vi "ME_acquire_11_DeltaForce.vi"() -> ()   [LabVIEW 2015]
doc: "Use this template to build a producer/consumer design pattern. Use this template when you need to execute a process, such as data analysis, when a data source, such as a triggered acquisition, produces data at an uneven rate and you need to execute the process when the data becomes available."
uses:
  Mode.ctl
  oxford_driver/Oxford Drivers/BUSGEN.LLB/OxfordAddress.ctl
  <vilib>/Analysis/baseanly.llb/Mean (DBL).vi
  <vilib>/Utility/file.llb/Write Delimited Spreadsheet (DBL).vi
  <vilib>/express/express arith-compare/Formula/XNode/ExpressFormulaBlockNode.xnode
  <vilib>/Analysis/NI_AALBase.lvlib
panel:
  in  "Averaged dt":dbl[][](array[numeric])
  in  "Averaged P(B)":dbl[][](array[numeric])
  out "LockInR":dbl
  out "deltaUaux":dbl
  out "Actual Voltage (V)":dbl caption="Actual AuxV" step=0.1
  out "remaining elements":T1(array[cluster])
  in  "Stop":bool
  out "SaveSweep":bool=TRUE
  out "Measurement File_dn":path
  out "Measurement File_up":path
  out "Measurement File_average":path
  out "Actual Polarization":dbl
  in  "Reset IB?":bool
  in  "First?":bool
  in  "Save Period":dbl=1.0
  out "Averaged I(B)":dbl[][](array[numeric])
  out "P(uC/mm^2)":dbl[](array[numeric])
  in  "Sweep":bool
  out "Offset array":dbl[](array[numeric])
  in  "stop 2":bool
  in  "dB":dbl=0.005
  in  "Dwell Time (ms)":u32=1
  out "appended array":dbl[][](array[numeric])
  out "Actual B Field (T)":dbl
  out "Actual Temperature (K)":dbl
  out "Actual Current (pA)":dbl
  in  "Tab Control":T2(tab)
  in  "Max temperature (K)":dbl=20.0
  in  "Min Temperature (K)":dbl=4.5
  out "P(T)":cluster{"yi":dbl[], dbl[]}(graph)
  out "I(T)":cluster{dbl[], dbl[]}(graph)
  in  "Set temperature (K)":dbl=4.5
  in  "Temp Ramping Rate (K/min)":dbl=10.0
  in  "Heater Range":enum16{"Off", "Low", "Medium", "High"}(ring)
  in  "Heater On/Off":bool
  out "Setpoint Temperature (K)":dbl
  in  "FileName":string
  out "Step Temp":bool
  out "j":i32
  out "i":i32
  in  "Max Countl":i32
  in  "Record ALL":bool
  in  "Sweep Rate Array":dbl[](array[numeric])=[2.0, 1.0, 0.5, 0.1, 0.05, 9.0, 10.0, 11.0, 12.0]
  out "I(B) 3":cluster{dbl[], dbl[]}[](graph)
  in  "Go to Set":bool
  in  "Set Field (T)":dbl
  in  "Field To Zero":bool
  in  "Sweep Rate (T/min)":dbl=2.0 format="%.6f"
  in  "Min Field (T)":dbl
  in  "Max Field (T)":dbl=0.15
  out "Up/Down":bool
  out "I(B) /Averaged/":cluster{"B array":dbl[], dbl[]}[](graph)
  in  "Temperature Array":dbl[](array[numeric])=[4.5, 5.0, 6.0, 7.0, 8.0, 9.0, 10.0, 11.0, 12.0]
  out "New":bool=TRUE
  out "Step Rate":bool
  out "Finished":bool=TRUE
  in  "Directory":string
  out "Wait (s)":dbl
  in  "secs to wait":dbl=180.0
  in  "Max count array":i32[](array[numeric])=[2, 1, 0, 0, 0, 9, 10, 11, 12]
  out "Target Field":dbl
  out "P(B) /Averaged/":cluster{"B array":dbl[], dbl[]}[](graph)
  out "P(B)":cluster{"yi":dbl[], dbl[]}(graph)
  in  "Measure Noise":bool
  in  "Cycles":i32
  in  "maximum value":dbl=10.0 format="%0.2f"
  in  "minimum value":dbl=-10.0 format="%0.2f"
  in  "physical channels":tag="Dev1/ai1"
  out "PSD (pA/Hz^1/2) Peaks Removed":cluster{"f0":dbl, "df":dbl, "magnitude":dbl[]}(graph)
  out "PSD (pA/Hz^1/2)":cluster{"f0":dbl, "df":dbl, "magnitude":dbl[]}(graph)
  out "Current (pA) Filtered":waveform(dbl)(graph)
  out "Current (pA)":dbl[](graph)
  in  "Samples per channel":i32=1000
  in  "Rate":dbl=1000.0 format="%0.2f"
  in  "Cut-Off Frequency":dbl=100.0 caption="Lower Cut-Off"
  in  "Filter On":bool
  in  "Lock_in_Amplifier":refnum<visa-resource-name>="GPIB0::5::INSTR"
  out "Dc offset":dbl
  in  "Calibrate":bool
  in  "IV converter":refnum<visa-resource-name>="GPIB0::20::INSTR"
  in  "Magnetic Field":refnum<visa-resource-name>="GPIB0::21::INSTR"
  out "Time Lag":dbl=0.0500025749206543
  in  "Lake Shore":refnum<visa-resource-name>="GPIB0::11::INSTR"
  in  "Temp Refresh (s)":dbl=0.1
  in  "Sampling rate (Hz)":dbl=10.0
  in  "Gain (V/A)":dbl=1000000000.0
  in  "Sample area (mm^2)":dbl=3.9
  out "B_V":cluster{dbl[], "Best Linear Fit":dbl[]}[](graph)=[{[-0.00854253601, 0.00626134724, 0.0219834428, 0.0379117736, 0.0535871506, 0.0694316728, 0.0851615152, 0.100816481, 0.116478038, 0.132148461, 0.147876163, 0.16341701, 0.178976744, 0.194563632, 0.210251739, 0.225738944, 0.241298253, 0.256806034, 0.272344374, 0.287933477, 0.303494709, 0.318997125, 0.334591297, 0.350146681, 0.365618053, 0.380940961, 0.39666457, 0.412213675, 0.427724671, 0.443221444, 0.458760641, 0.474360042, 0.489915118, 0.505330598, 0.520967119, 0.536347531, 0.551813711, 0.567441155, 0.582995861, 0.598507522, 0.614041988, 0.629563151, 0.645106262, 0.660611914, 0.676136149, 0.691553948, 0.7071244, 0.72262999, 0.738171137, 0.753700392, 0.76919513, 0.784778028, 0.800215944, 0.8156961, 0.831325434, 0.846852183, 0.862326812, 0.877819169, 0.893312568, 0.90888536, 0.924354789], "Best Linear Fit"=[0.0, 0.005, 0.01, 0.015, 0.02, 0.025, 0.03, 0.035, 0.04, 0.045, 0.05, 0.055, 0.06, 0.065, 0.07, 0.075, 0.08, 0.085, 0.09, 0.095, 0.1, 0.105, 0.11, 0.115, 0.12, 0.125, 0.13, 0.135, 0.14, 0.145, 0.15, 0.155, 0.16, 0.165, 0.17, 0.175, 0.18, 0.185, 0.19, 0.195, 0.2, 0.205, 0.21, 0.215, 0.22, 0.225, 0.23, 0.235, 0.24, 0.245, 0.25, 0.255, 0.26, 0.265, 0.27, 0.275, 0.28, 0.285, 0.29, 0.295, 0.3]}, {[-0.00854253601, 0.00626134724, 0.0219834428, 0.0379117736, 0.0535871506, 0.0694316728, 0.0851615152, 0.100816481, 0.116478038, 0.132148461, 0.147876163, 0.16341701, 0.178976744, 0.194563632, 0.210251739, 0.225738944, 0.241298253, 0.256806034, 0.272344374, 0.287933477, 0.303494709, 0.318997125, 0.334591297, 0.350146681, 0.365618053, 0.380940961, 0.39666457, 0.412213675, 0.427724671, 0.443221444, 0.458760641, 0.474360042, 0.489915118, 0.505330598, 0.520967119, 0.536347531, 0.551813711, 0.567441155, 0.582995861, 0.598507522, 0.614041988, 0.629563151, 0.645106262, 0.660611914, 0.676136149, 0.691553948, 0.7071244, 0.72262999, 0.738171137, 0.753700392, 0.76919513, 0.784778028, 0.800215944, 0.8156961, 0.831325434, 0.846852183, 0.862326812, 0.877819169, 0.893312568, 0.90888536, 0.924354789], "Best Linear Fit"=[-0.00022554388023060128, 0.004536267537808887, 0.009593430775915074, 0.014716931562355689, 0.01975906732634002, 0.024855610270593523, 0.029915265354287977, 0.03495083565949541, 0.03998852608757118, 0.045029068349812316, 0.05008803495326229, 0.055086897848955874, 0.060091835929837946, 0.06510550835596321, 0.07015173884687344, 0.07513334727738563, 0.08013814865293042, 0.08512637555172443, 0.0901244320467579, 0.09513881694893507, 0.10014423687592358, 0.10513073807087174, 0.11014675346564809, 0.1151502923271957, 0.12012680792099008, 0.1250555686413888, 0.1301132186920259, 0.13511473785283767, 0.14010399888730068, 0.14508868495702945, 0.1500870171143548, 0.15510471446726903, 0.16010815425765457, 0.16506669165212906, 0.17009632901003072, 0.1750435864450521, 0.18001843198211442, 0.1850451496356715, 0.19004847041199868, 0.1950379453501071, 0.20003475573578386, 0.20502728708357412, 0.21002687821664084, 0.21501442030211, 0.220007939788244, 0.2249672231113706, 0.22997560874002893, 0.23496313088260184, 0.23996209027618054, 0.24495722449359253, 0.24994125598600042, 0.2549536449902534, 0.25991939913989753, 0.2648987401917687, 0.26992606578200207, 0.2749203939204135, 0.2798979571595809, 0.2848812227804405, 0.2898648235706211, 0.2948739618827834, 0.2998498524919418]}]
  out "V_I":cluster{dbl[], "Best Linear Fit":dbl[]}[](graph)=[{[0.0, 0.035, 0.069, 0.104, 0.138, 0.173, 0.208, 0.242, 0.277, 0.311, 0.346, 0.38, 0.415, 0.45, 0.484, 0.519, 0.553, 0.588, 0.623, 0.657, 0.692, 0.726, 0.761, 0.796, 0.83, 0.865, 0.899, 0.934, 0.969, 1.003, 1.038, 1.072, 1.107, 1.141, 1.176, 1.211, 1.245, 1.28, 1.314, 1.349, 1.384, 1.418, 1.453, 1.487, 1.522, 1.557, 1.591, 1.626, 1.66, 1.695, 1.73, 1.764, 1.799, 1.833, 1.868, 1.902, 1.937, 1.972, 2.006, 2.041, 2.075], "Best Linear Fit"=[-0.00854253601, 0.00626134724, 0.0219834428, 0.0379117736, 0.0535871506, 0.0694316728, 0.0851615152, 0.100816481, 0.116478038, 0.132148461, 0.147876163, 0.16341701, 0.178976744, 0.194563632, 0.210251739, 0.225738944, 0.241298253, 0.256806034, 0.272344374, 0.287933477, 0.303494709, 0.318997125, 0.334591297, 0.350146681, 0.365618053, 0.380940961, 0.39666457, 0.412213675, 0.427724671, 0.443221444, 0.458760641, 0.474360042, 0.489915118, 0.505330598, 0.520967119, 0.536347531, 0.551813711, 0.567441155, 0.582995861, 0.598507522, 0.614041988, 0.629563151, 0.645106262, 0.660611914, 0.676136149, 0.691553948, 0.7071244, 0.72262999, 0.738171137, 0.753700392, 0.76919513, 0.784778028, 0.800215944, 0.8156961, 0.831325434, 0.846852183, 0.862326812, 0.877819169, 0.893312568, 0.90888536, 0.924354789]}, {[0.0, 0.035, 0.069, 0.104, 0.138, 0.173, 0.208, 0.242, 0.277, 0.311, 0.346, 0.38, 0.415, 0.45, 0.484, 0.519, 0.553, 0.588, 0.623, 0.657, 0.692, 0.726, 0.761, 0.796, 0.83, 0.865, 0.899, 0.934, 0.969, 1.003, 1.038, 1.072, 1.107, 1.141, 1.176, 1.211, 1.245, 1.28, 1.314, 1.349, 1.384, 1.418, 1.453, 1.487, 1.522, 1.557, 1.591, 1.626, 1.66, 1.695, 1.73, 1.764, 1.799, 1.833, 1.868, 1.902, 1.937, 1.972, 2.006, 2.041, 2.075], "Best Linear Fit"=[-0.007846580254753975, 0.007882153481927697, 0.02316149482613275, 0.03889022856281441, 0.054169569907019474, 0.06989830364370113, 0.08562703738038281, 0.10090637872458785, 0.11663511246126955, 0.1319144538054746, 0.14764318754215625, 0.1629225288863613, 0.17865126262304296, 0.19437999635972467, 0.2096593377039297, 0.22538807144061138, 0.24066741278481643, 0.25639614652149806, 0.27212488025817977, 0.2874042216023848, 0.3031329553390665, 0.31841229668327153, 0.3341410304199532, 0.3498697641566349, 0.3651491055008399, 0.3808778392375216, 0.39615718058172666, 0.4118859143184083, 0.42761464805509, 0.442893989399295, 0.45862272313597674, 0.4739020644801818, 0.48963079821686345, 0.5049101395610684, 0.5206388732977502, 0.5363676070344319, 0.5516469483786369, 0.5673756821153185, 0.5826550234595236, 0.5983837571962053, 0.6141124909328869, 0.629391832277092, 0.6451205660137737, 0.6603999073579787, 0.6761286410946604, 0.691857374831342, 0.7071367161755471, 0.7228654499122288, 0.7381447912564338, 0.7538735249931156, 0.7696022587297972, 0.7848816000740022, 0.8006103338106839, 0.815889675154889, 0.8316184088915707, 0.8468977502357756, 0.8626264839724573, 0.878355217709139, 0.893634559053344, 0.9093632927900257, 0.9246426341342309]}]
  out "B0 (T)":dbl=0.0025222449819540214
  out "B/V (T/V)":dbl=0.321659617116981
  out "I0 (A)":dbl=-0.007846580254753975
  out "V/I (Ohm)":dbl=0.44939239247661916
  in  "Offset?":bool
  in  "Magnet":bool
  in  "Ramp":bool=TRUE
  in  "Temp/Magnetic Field":bool
  out "index":i8
  out "Read?":bool
  out "Magnetic Field (T)":dbl[](array[numeric])
  out "Reset":bool
  out "Measured Current (pA)":dbl[](array[numeric])
  out "Elapsed Time (s)":dbl[](array[numeric])
  out "Start time":timestamp
  in  "Enum":T3=enum."Process"
  out "B array":dbl[](array[numeric])
  in  "dB (T)":dbl=0.0025
  in  "Counter":i8
  out "L magnet (H)":dbl
  out "R magnet (mOhm)":dbl
  out "Actual Current (R0)":dbl
  out "Actual Field (T)":dbl
  out "Temperature array":dbl[](array[numeric])
  in  "New Measurement File":bool
  out "Measurement File":path
  out "refnum out":refnum<file>
  in  "Measuring":bool
  in  "Measure /Pause":bool
  in  "stop":bool
  # "DeltaForce"
  # "Discrete"
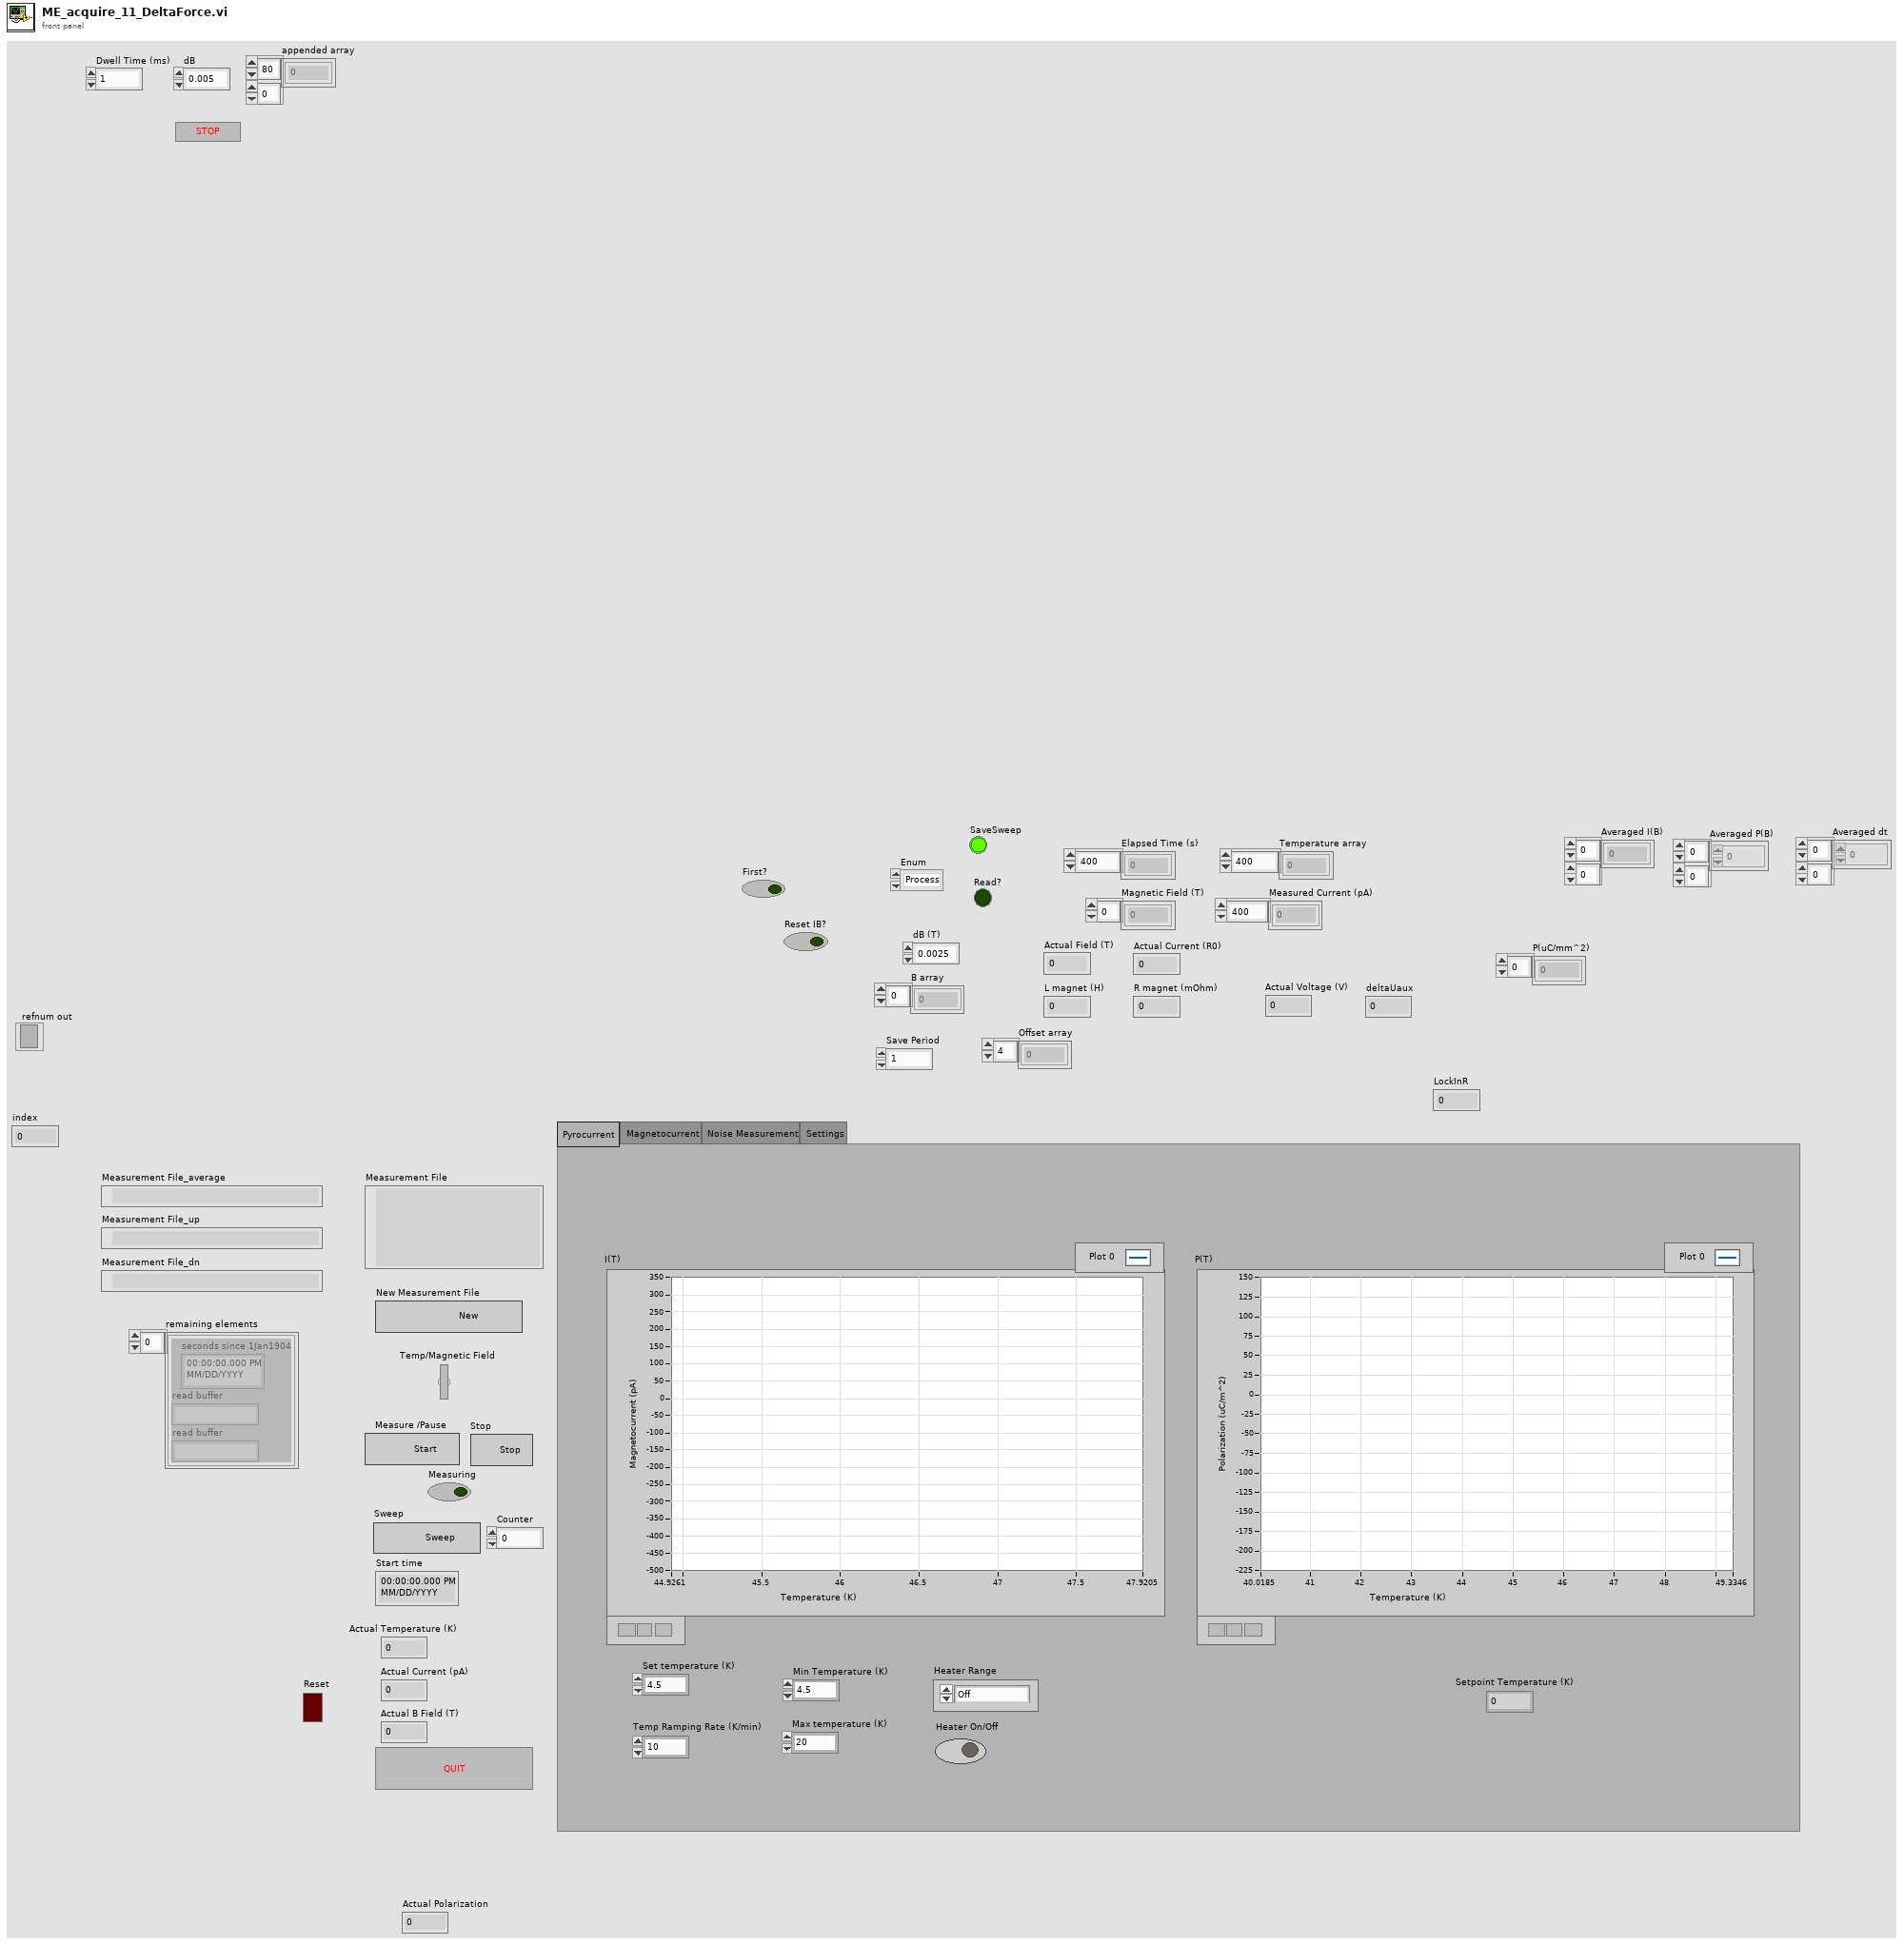
[diagram p1: front panel]
types:
  T1 = cluster{"seconds since 1Jan1904":timestamp, "read buffer":string, "read buffer":string}[]
  T2 = enum32{"Pyrocurrent", "Magnetocurrent", "Noise Measurement", "Settings"}
  T3 = typedef "Mode.ctl" = enum16{"Offset", "Process", "Sweep", "StepField", "Plot", "Save", "New", "Return", ""}
  T4 = enum16{"open", "replace", "create", "open or create", "replace or create", "replace or create with confirmation"}
  T5 = typedef "OxfordAddress.ctl" = cluster{"Com Port":i32, "ISOBUS Address":i32, "GPIB Address":i16, "Communication":enum16{"RS232", "ISOBUS", "GPIB", "Gateway"}}
  T6 = cluster{"seconds since 1Jan1904":timestamp, "read buffer":string, "read buffer":string}
  T7 = cluster{"B array":dbl[], "Averaged P(B) Out":dbl[]}
  T8 = cluster{"B array":dbl[], "Averaged I(B) out":dbl[]}
  T9 = cluster{"B array":dbl[], "Averaged P(B) Out":dbl[]}[]
  T10 = cluster{"B array":dbl[], "Averaged I(B) out":dbl[]}[]
  T11 = cluster{"I array out (A)":dbl[], "V array out (V)":dbl[]}
  T12 = cluster{"I array out (A)":dbl[], "Best Linear Fit":dbl[]}
  T13 = cluster{"V array out (V)":dbl[], "B array Out":dbl[]}
  T14 = cluster{"V array out (V)":dbl[], "Best Linear Fit 2":dbl[]}
  T15 = cluster{"I array out (A)":dbl[], "Best Linear Fit":dbl[]}[]
  T16 = cluster{"V array out (V)":dbl[], "Best Linear Fit 2":dbl[]}[]
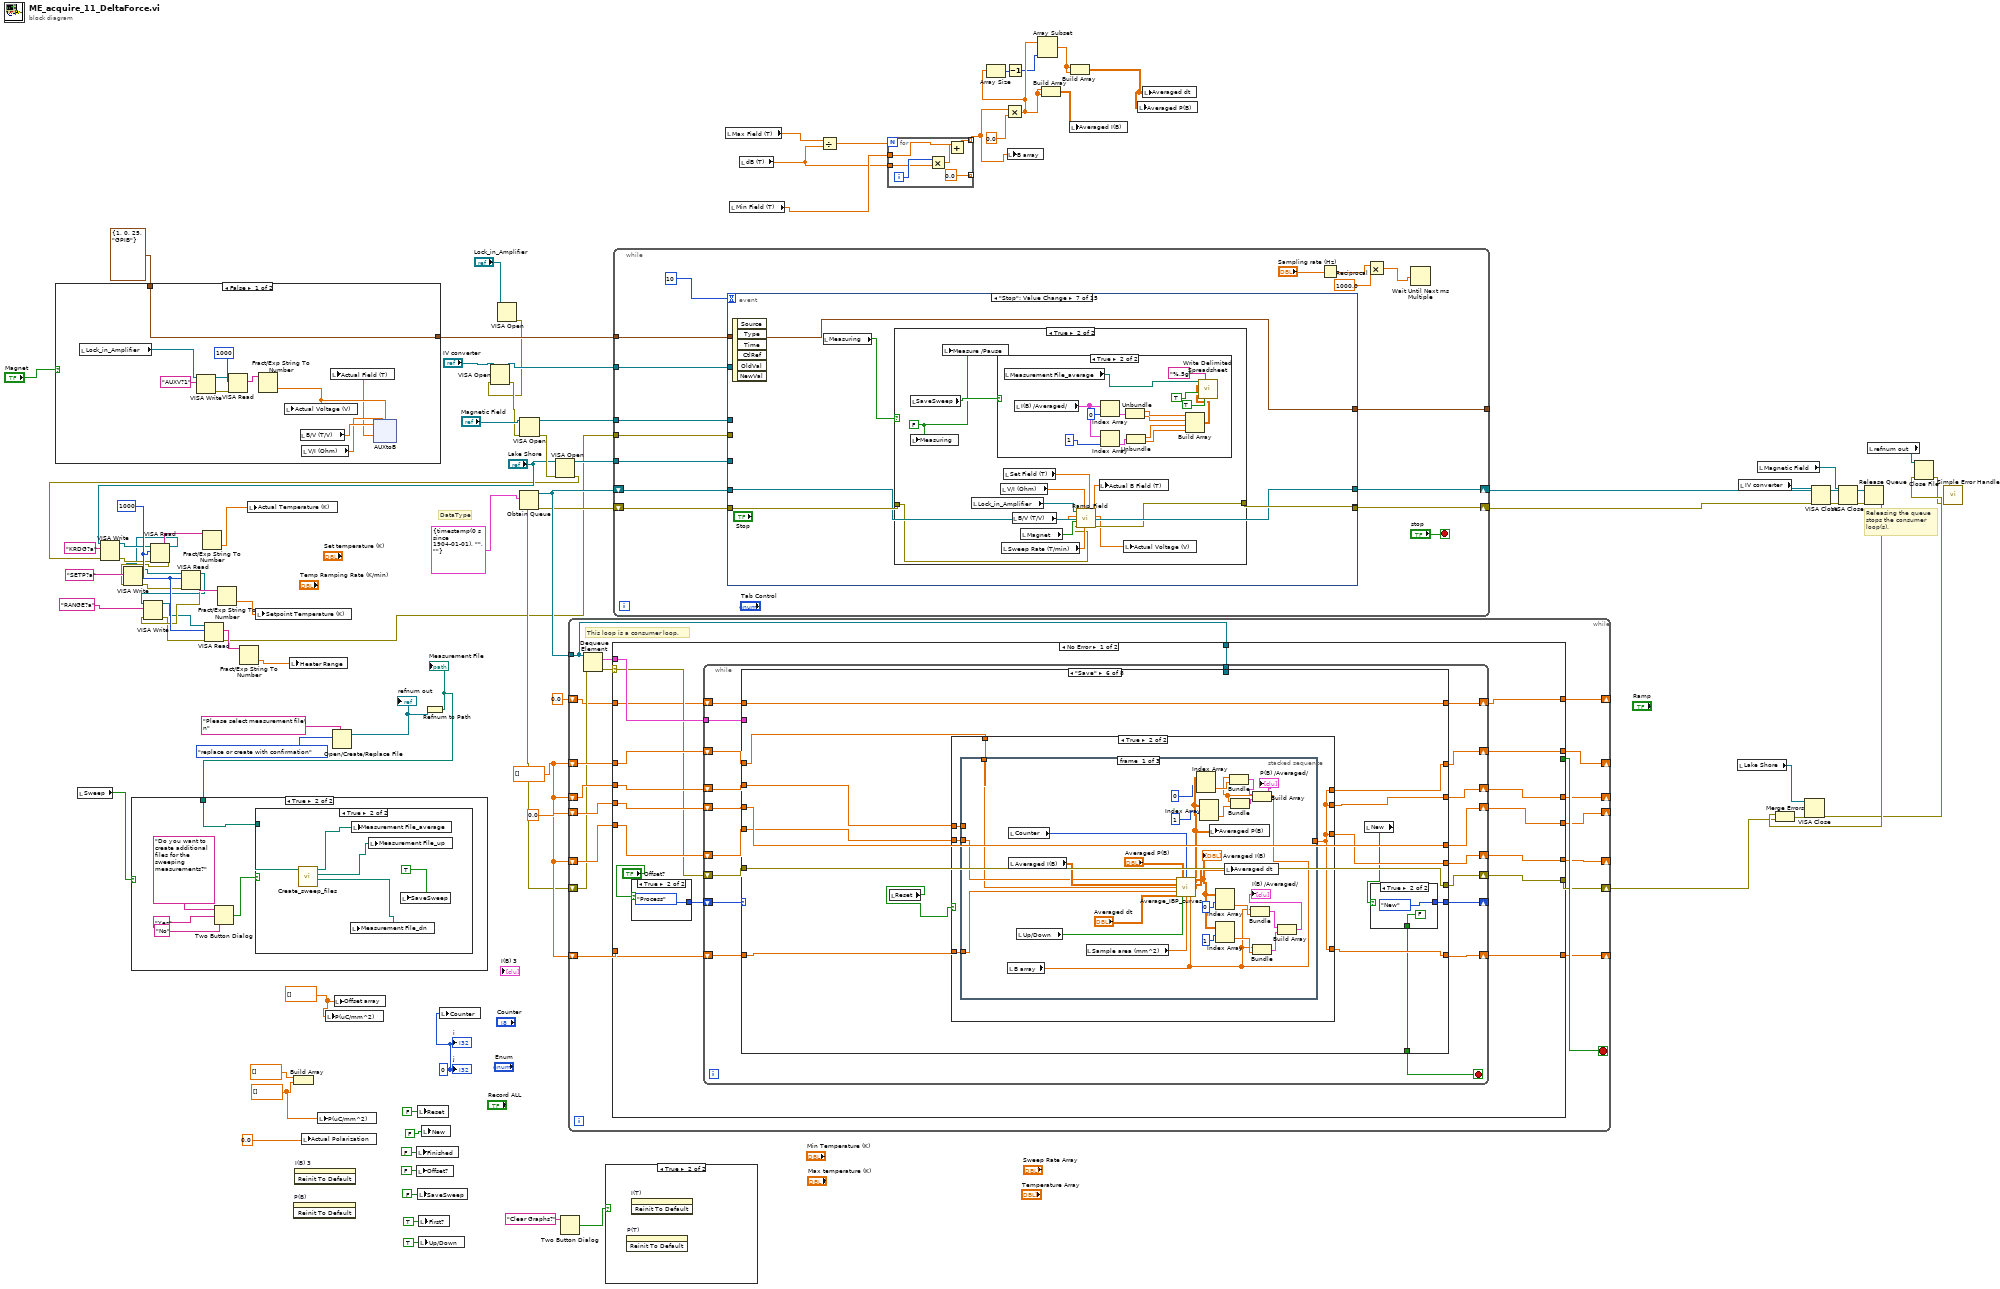
[diagram p0: block diagram]
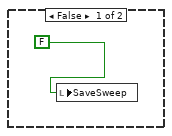
[diagram p4: hidden frame]
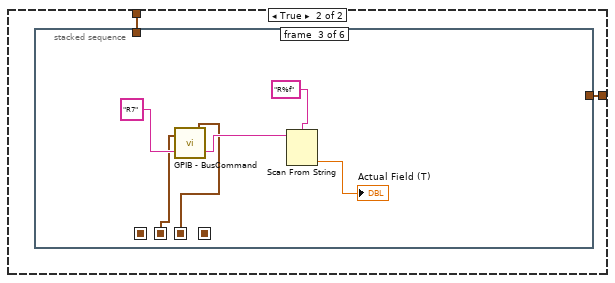
[diagram p5: hidden frame]
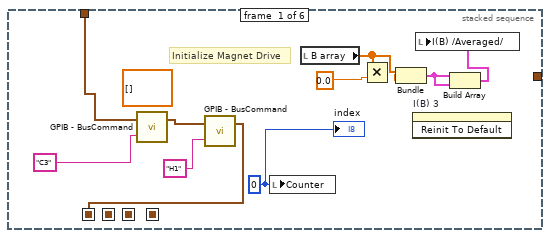
[diagram p6: hidden frame]
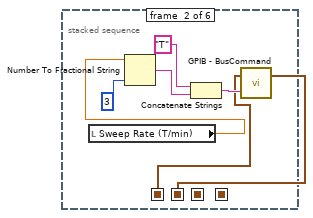
[diagram p7: hidden frame]
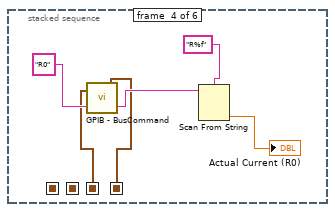
[diagram p8: hidden frame]
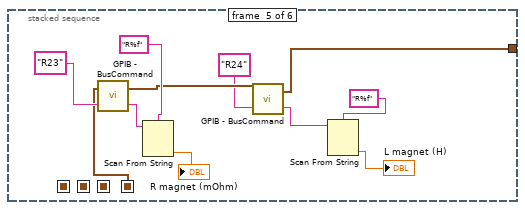
[diagram p9: hidden frame]
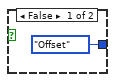
[diagram p11: hidden frame]
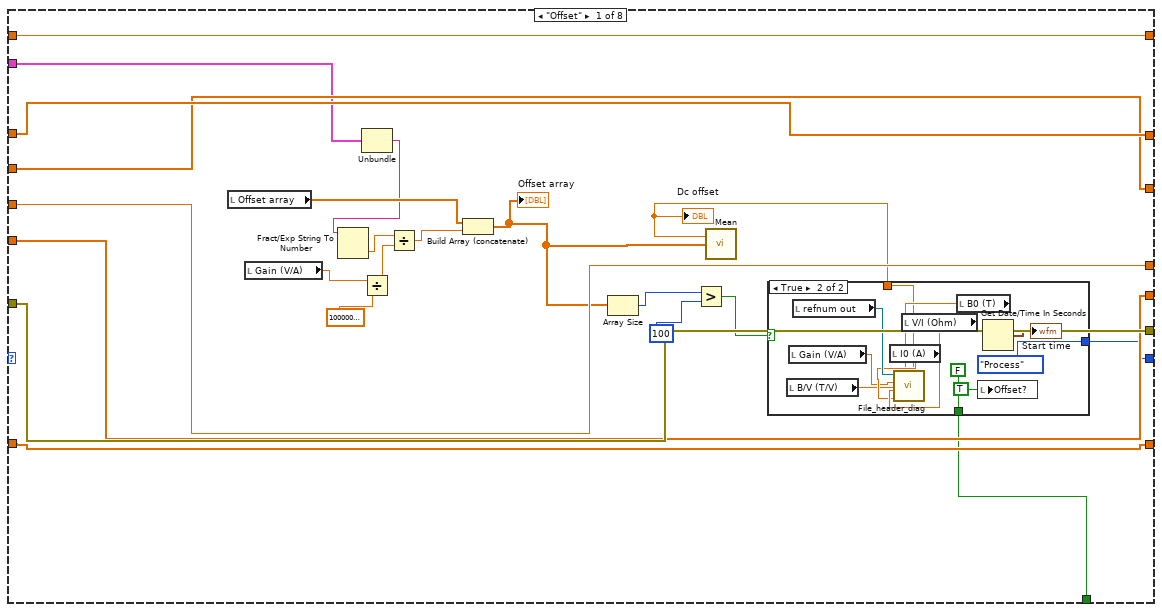
[diagram p12: hidden frame]
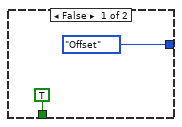
[diagram p13: hidden frame]
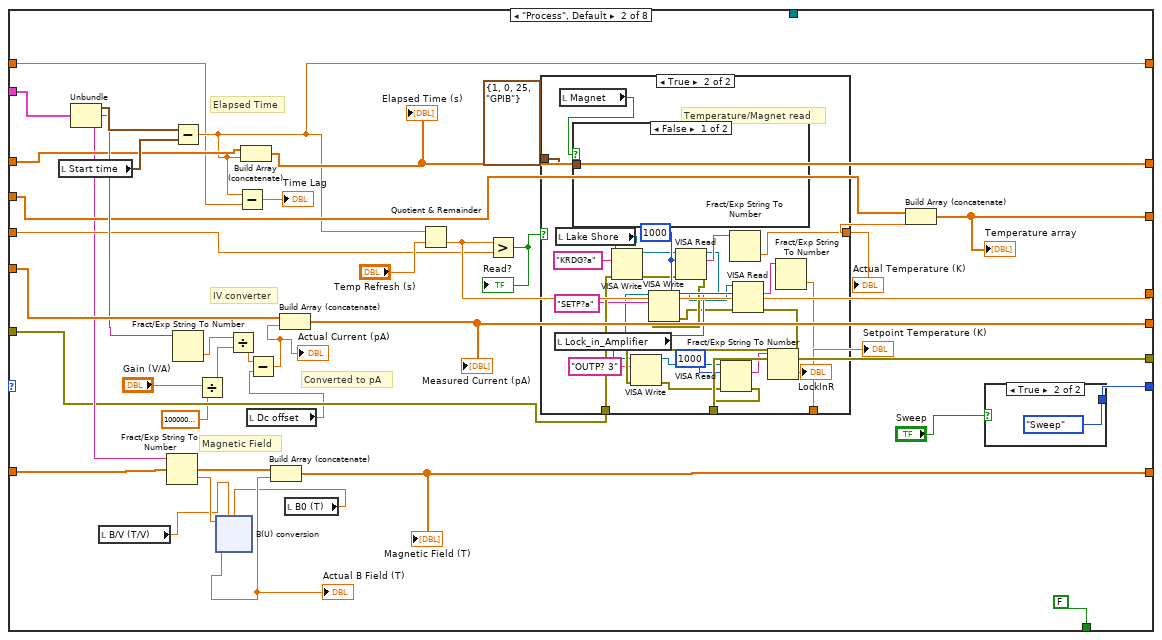
[diagram p14: hidden frame]
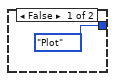
[diagram p15: hidden frame]
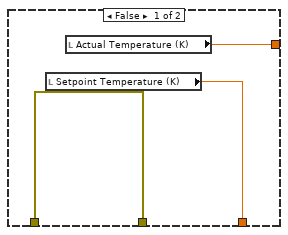
[diagram p16: hidden frame]
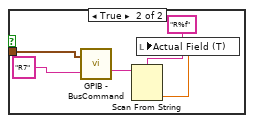
[diagram p17: hidden frame]
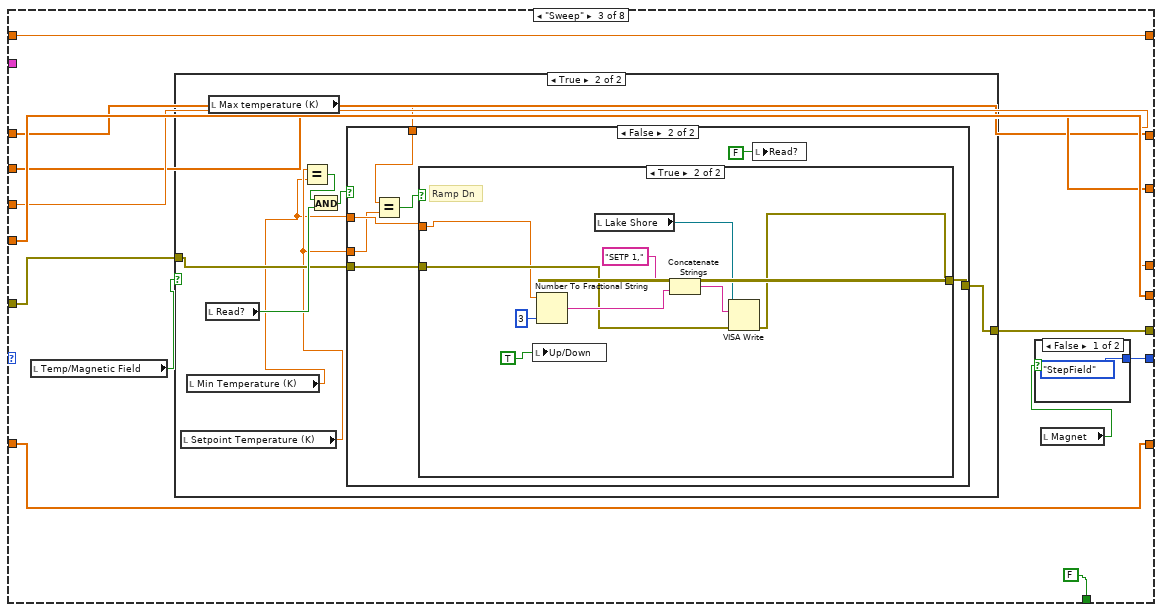
[diagram p18: hidden frame]
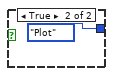
[diagram p19: hidden frame]
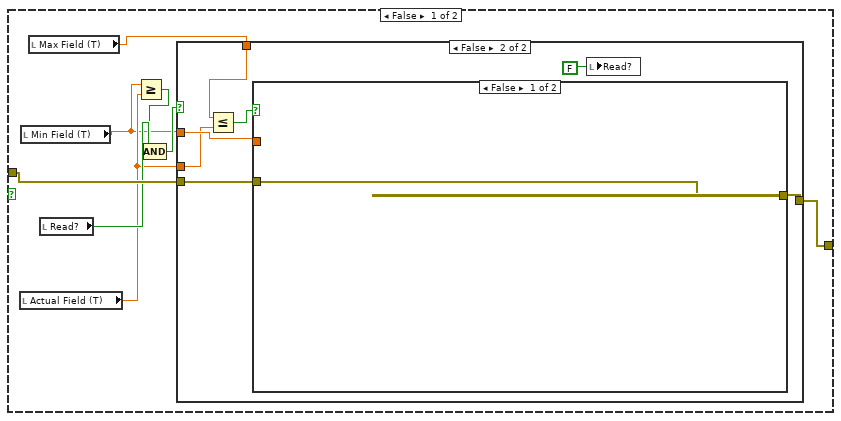
[diagram p20: hidden frame]
diagram:
  w27 = u32 1000 ("byte count")
  w38 = 0 ("j")
  w35 = dbl[] []
  w53 = dbl[] []
  w59 = dbl[] []
  # "DataType"
  # "Releasing the queue stops the consumer loop(s)."
  n1 = case shown="False" "Magnet" {
    tunnel: T5 {"Com Port"=1, "ISOBUS Address"=0, "GPIB Address"=25, "Communication"=enum."GPIB"} ("Address") -> [w96 w110]
    tunnel: [w96 w109] -> w65
    frame False {
      n2 = local read "Lock_in_Amplifier"() -> (w90:refnum<visa-resource-name>)
      n3 = VISA Write(VISA resource name=w90, write buffer="AUXV?1") -> (VISA resource name out=w91:refnum<visa-resource-name>, error out=w95:errorcluster)  [unwired: 1 in, 1 out]
      n4 = VISA Read(VISA resource name=w91, byte count=u32 1000, error in (no error)=w95) -> (read buffer=w94:string)  [unwired: 3 out]
      n5 = Fract/Exp String To Number(string=w94) -> (number=w87:dbl)  [unwired: 3 in, 1 out]
      n6 = local write "Actual Voltage (V)"(w87) -> ()
      n7 = local read "B/V (T/V)"() -> (w89:dbl)
      n8 = local read "V/I (Ohm)"() -> (w88:dbl)
      n9 = xnode "AUXtoB"("BpV"=w89, "Rm"=w88, "Aux"=w87) -> ("Result"=w86:dbl)  [unwired: 1 in, 1 out]
      n10 = local write "Actual Field (T)"(w86) -> ()
    }
    frame True {
      n11 = stacked-sequence {
        seq-local: [w118 _ _ _ _ _] -> [_ w123 _ _ _ _]
        seq-local: [_ w122 _ _ _ _] -> [_ _ w130 _ _ _]
        seq-local: [_ _ w129 _ _ _] -> [_ _ _ w136 _ _]
        seq-local: [_ _ _ w135 _ _] -> [_ _ _ _ w147 _]
        tunnel: w110 -> [w120 _ _ _ _ _]
        tunnel: [_ _ _ _ w145 _] -> w109
        frame #0 {
          (unwired) dbl[][] []
          w116 = i8 0 ("Counter")
          # "Initialize Magnet Drive"
          n12 = call "GPIB - BusCommand.vi"("Command"="C3", "Address"=w120) -> ("Address(thru)"=w119:T5)  [unwired: 1 out]
          n13 = call "GPIB - BusCommand.vi"("Command"="H1", "Address"=w119) -> ("Address(thru)"=w118:T5)  [unwired: 1 out]
          n14 = local write "Counter"(w116) -> ()
          n15 = local read "B array"() -> (w114:dbl[])
          n16 = Multiply(x=w114, y=0.0) -> (x*y=w113:dbl[])
          n17 = Bundle("B array"=w114, w113) -> (w112:cluster{"B array":dbl[], dbl[]})  [unwired: 1 in]
          n18 = invoke on="I(B) 3" class="XYGraph (strict)" method="Reinit To Default"() -> ()  [unwired: 3 in, 3 out]
          n19 = Build Array(w112, w112) -> (w111:cluster{"B array":dbl[], dbl[]}[])
          n20 = local write "I(B) /Averaged/"(w111) -> ()
          "index" <- w116
        }
        frame #1 {
          n21 = local read "Sweep Rate (T/min)"() -> (w124:dbl)
          n22 = Number To Fractional String(number=w124, precision (6)=i16 3) -> (F-format string=w126:string)  [unwired: 2 in]
          n23 = Concatenate Strings("T" ("format string"), w126) -> (w125:string)
          n24 = call "GPIB - BusCommand.vi"("Command"=w125, "Address"=w123) -> ("Address(thru)"=w122:T5)  [unwired: 1 out]
        }
        frame #2 {
          n25 = call "GPIB - BusCommand.vi"("Command"="R7" ("format string"), "Address"=w130) -> ("Reply"=w134:string, "Address(thru)"=w129:T5)
          n26 = Scan From String(format string="R%f" ("remaining string"), input string=w134) -> (output 1=→"Actual Field (T)":dbl)  [unwired: 3 in, 3 out]
        }
        frame #3 {
          n27 = call "GPIB - BusCommand.vi"("Command"="R0" ("format string"), "Address"=w136) -> ("Reply"=w140:string, "Address(thru)"=w135:T5)
          n28 = Scan From String(format string="R%f" ("remaining string"), input string=w140) -> (output 1=→"Actual Current (R0)":dbl)  [unwired: 3 in, 3 out]
        }
        frame #4 {
          n29 = call "GPIB - BusCommand.vi"("Command"="R23" ("format string"), "Address"=w147) -> ("Reply"=w151:string, "Address(thru)"=w146:T5)
          n30 = Scan From String(format string="R%f" ("remaining string"), input string=w151) -> (output 1=→"R magnet (mOhm)":dbl)  [unwired: 3 in, 3 out]
          n31 = call "GPIB - BusCommand.vi"("Command"="R24" ("format string"), "Address"=w146) -> ("Reply"=w143:string, "Address(thru)"=w145:T5)
          n32 = Scan From String(format string="R%f" ("remaining string"), input string=w143) -> (output 1=→"L magnet (H)":dbl)  [unwired: 3 in, 3 out]
        }
        frame #5 {
        }
      }
    }
  }
  n33 = local read "Sweep"() -> (w43:bool)
  n34 = Build Array(dbl[] [], w35) -> ()  [unwired: 1 out]
  n35 = invoke on="P(B)" class="XYGraph (strict)" method="Reinit To Default"() -> ()  [unwired: 3 in, 3 out]
  n36 = invoke on="I(B) 3" class="XYGraph (strict)" method="Reinit To Default"() -> ()  [unwired: 3 in, 3 out]
  n37 = local write "Actual Polarization"(0.0 ("Actual Polarization")) -> ()
  n38 = local write "P(uC/mm^2)"(w35) -> ()
  n39 = local write "P(uC/mm^2)"(w53) -> ()
  n40 = Open/Create/Replace File(prompt="Please select measurement file\n", operation (0:open)=T4."replace or create with confirmation") -> (refnum out=w62:refnum<file>)  [unwired: 4 in, 2 out]
  "refnum out" <- w62
  n41 = local write "Offset array"(w53) -> ()
  n42 = local write "Finished"(FALSE ("Finished")) -> ()
  n43 = local write "Offset?"(FALSE ("Offset?")) -> ()
  n44 = local write "Reset"(FALSE ("Reset")) -> ()
  n45 = local write "SaveSweep"(FALSE ("SaveSweep")) -> ()
  n46 = local write "First?"(TRUE ("First?")) -> ()
  n47 = local write "Up/Down"(TRUE ("Up/Down")) -> ()
  n48 = local write "New"(FALSE ("New")) -> ()
  n49 = Refnum to Path(1:w62) -> (0:w42:path)
  "Measurement File" <- w42
  n50 = case shown="True" w43 {
    tunnel: w42 -> [_ w152]
    frame False {
    }
    frame True {
      n51 = Two Button Dialog(message="Do you want to create additional files for the sweeping measurements?" ("string"), 1:"No" ("F button name (\"Cancel\")"), 2:"Yes" ("T button name (\"OK\")")) -> (T button?=w154:bool)
      n52 = case shown="True" w154 {
        tunnel: w152 -> [_ w162]
        frame False {
          n53 = local write "SaveSweep"(FALSE ("SaveSweep")) -> ()
        }
        frame True {
          n54 = call "Create_sweep_files.vi"("Measurement File"=w162) -> ("Path 3"=w159:path, "Path 2"=w160:path, "Path"=w161:path)  [unwired: 8 in]
          n55 = local write "Measurement File_dn"(w159) -> ()
          n56 = local write "Measurement File_average"(w161) -> ()
          n57 = local write "Measurement File_up"(w160) -> ()
          n58 = local write "SaveSweep"(TRUE) -> ()
        }
      }
    }
  }
  n59 = local write "Counter"(w38) -> ()
  n60 = VISA Open(VISA resource name="Lock_in_Amplifier") -> (error out=w10:errorcluster)  [unwired: 4 in, 1 out]
  n61 = VISA Open(error in (no error)=w10, VISA resource name="IV converter") -> (VISA resource name=w80:refnum<visa-resource-name>, error out=w82:errorcluster)  [unwired: 3 in]
  n62 = Obtain Queue(element data type=T6 {"seconds since 1Jan1904"=timestamp(0 s since 1904-01-01), "read buffer"="", "read buffer"=""} ("output cluster")) -> (queue out=w85:refnum<queue>, error out=w57:errorcluster)  [unwired: 4 in, 1 out]
  n63 = VISA Open(error in (no error)=w82, VISA resource name="Magnetic Field") -> (VISA resource name=w79:refnum<visa-resource-name>, error out=w60:errorcluster)  [unwired: 3 in]
  n64 = VISA Open(error in (no error)=w60, VISA resource name="Lake Shore") -> (VISA resource name=w55:refnum<visa-resource-name>, error out=w24:errorcluster)  [unwired: 3 in]
  n65 = VISA Write(VISA resource name="Lake Shore", write buffer="KRDG?a", error in (no error)=w24) -> (VISA resource name out=w21:refnum<visa-resource-name>, error out=w20:errorcluster)  [unwired: 1 out]
  n66 = VISA Read(VISA resource name=w21, byte count=w27, error in (no error)=w20) -> (VISA resource name out=w18:refnum<visa-resource-name>, read buffer=w32:string, error out=w19:errorcluster)  [unwired: 1 out]
  n67 = VISA Write(VISA resource name=w18, write buffer="SETP?a", error in (no error)=w19) -> (VISA resource name out=w17:refnum<visa-resource-name>, error out=w16:errorcluster)  [unwired: 1 out]
  n68 = VISA Read(VISA resource name=w17, byte count=w27, error in (no error)=w16) -> (VISA resource name out=w14:refnum<visa-resource-name>, read buffer=w31:string, error out=w15:errorcluster)  [unwired: 1 out]
  n69 = VISA Write(VISA resource name=w14, write buffer="RANGE?a", error in (no error)=w15) -> (VISA resource name out=w12:refnum<visa-resource-name>, error out=w13:errorcluster)  [unwired: 1 out]
  n70 = Fract/Exp String To Number(string=w32) -> (number=w30:dbl)  [unwired: 3 in, 1 out]
  n71 = VISA Read(VISA resource name=w12, byte count=w27, error in (no error)=w13) -> (read buffer=w26:string, error out=w23:errorcluster)  [unwired: 2 out]
  n72 = Fract/Exp String To Number(string=w31) -> (number=w29:dbl)  [unwired: 3 in, 1 out]
  n73 = Fract/Exp String To Number(string=w26) -> (number=w22:dbl)  [unwired: 3 in, 1 out]
  n74 = local write "Actual Temperature (K)"(w30) -> ()
  n75 = local write "Setpoint Temperature (K)"(w29) -> ()
  n76 = local write "Heater Range"(w22) -> ()
  n77 = Two Button Dialog(message="Clear Graphs?") -> (T button?=w37:bool)  [unwired: 2 in]
  n78 = while {
    tunnel: w85 -> [w163]
    shift-right: [w176] -> _
    shift-left: w59 -> [w175]
    shift-right: [w174] -> _
    shift-left: w59 -> [w173]
    shift-right: [w172] -> _
    shift-left: w59 -> [w171]
    shift-right: [w170] -> _
    shift-left: 0.0 -> [w169]
    shift-right: [w168] -> _
    shift-left: w59 -> [w167]
    shift-right: [w177] -> w70
    shift-left: w57 -> [w166]
    shift-right: [w165] -> _
    shift-left: 0.0 -> [w164]
    stop <- w178 stop-if-true
    # "This loop is a consumer loop."
    n79 = Dequeue Element(queue=w163, error in (no error)=w166) -> (element=w179:T6, error out=w180:errorcluster)  [unwired: 1 in, 2 out]
    n80 = case shown="No Error" w180 {
      selector: w180 -> [w186 w841]
      tunnel: w179 -> [w197 _]
      tunnel: [_ TRUE] -> w178
      tunnel: [w185 w841] -> w177
      tunnel: [w196 w840] -> w176
      tunnel: w175 -> [w195 w840]
      tunnel: [w194 w837] -> w174
      tunnel: w173 -> [w193 w837]
      tunnel: [w192 w836] -> w172
      tunnel: w171 -> [w191 w836]
      tunnel: [w190 w838] -> w170
      tunnel: w169 -> [w189 w838]
      tunnel: [w188 w839] -> w168
      tunnel: w167 -> [w187 w839]
      tunnel: [w184 w835] -> w165
      tunnel: w164 -> [w183 w835]
      tunnel: w163 -> [w181 _]
      frame No Error {
        n81 = case shown="True" "Offset?" {
          tunnel: [Mode."Offset" ("Enum") Mode."Process" ("Enum")] -> w198
          frame False {
          }
          frame True {
          }
        }
        n82 = while {
          shift-right: [w207] -> _
          shift-left: w198 -> [w219]
          tunnel: w197 -> [w218]
          shift-right: [w217] -> w196
          shift-left: w195 -> [w216]
          shift-right: [w209] -> w188
          shift-left: w187 -> [w208]
          shift-right: [w211] -> w190
          shift-left: w189 -> [w210]
          shift-right: [w215] -> w194
          shift-left: w193 -> [w214]
          shift-right: [w205] -> w185
          shift-left: w186 -> [w206]
          shift-right: [w213] -> w192
          shift-left: w191 -> [w212]
          shift-right: [w203] -> w184
          shift-left: w183 -> [w202]
          tunnel: w181 -> [w201]
          stop <- w204 stop-if-true
          n83 = case shown="\"Save\"" w219 {
            selector: w219 -> [_ _ _ _ _ _ _ w828]
            tunnel: w218 -> [w235 w291 _ _ _ _ _ _]
            tunnel: [w241 w288 w346 w461 w523 w596 w677 w833] -> w217
            tunnel: w216 -> [w241 w279 w346 w461 w523 w592 w677 w833]
            tunnel: [w236 w287 w349 w458 w525 w598 w675 w830] -> w215
            tunnel: w214 -> [w236 w286 w349 w458 w525 w593 w675 w830]
            tunnel: [w237 w283 w351 w456 w520 w599 w673 w827] -> w213
            tunnel: w212 -> [w237 w282 w351 w456 w520 w594 w673 w827]
            tunnel: [w239 w278 w348 w459 w521 w602 0.0 w831] -> w211
            tunnel: w210 -> [w239 w277 w348 w459 w521 w602 _ w831]
            tunnel: [w240 w274 w347 w460 w522 w597 w676 w832] -> w209
            tunnel: w208 -> [w240 w275 w347 w460 w522 w595 w676 w832]
            tunnel: [w224 w272 w344 Mode."Plot" ("Enum") Mode."Save" ("Enum") w603 Mode."Return" ("Enum") w828] -> w207
            tunnel: w206 -> [w238 w270 w353 w453 w528 w601 w669 w829]
            tunnel: [w238 w269 w352 w452 w528 w601 w668 w829] -> w205
            tunnel: [w220 FALSE FALSE FALSE FALSE w590 TRUE TRUE] -> w204
            tunnel: [w223 w266 w345 w454 w524 w600 0.0 w834] -> w203
            tunnel: w202 -> [w223 w265 w345 w454 w524 w600 _ w834]
            tunnel: w201 -> [_ _ _ _ _ _ w667 _]
            frame "Offset" {
              n84 = local read "Offset array"() -> (w229:dbl[])
              n85 = local read "Gain (V/A)"() -> (w233:dbl)
              n86 = Unbundle(w235) -> ("read buffer"=w222:string)  [unwired: 2 out]
              n87 = Fract/Exp String To Number(string=w222) -> (number=w234:dbl)  [unwired: 3 in, 1 out]
              n88 = Divide(x=w233, y=1000000000000.0) -> (x/y=w231:dbl)
              n89 = Divide(x=w234, y=w231) -> (x/y=w230:dbl)
              n90 = Build Array (concatenate)(w229, w230) -> (w225:dbl[])
              "Offset array" <- w225
              n91 = Array Size(array=w225) -> (size(s)=w228:i32)
              n92 = Greater?(x=w228, y=100) -> (0:w226:bool)
              n93 = call-poly <vilib>:"Mean.vi"("X"=w225) -> ("mean"=w221:dbl)  [unwired: 1 out]
              "Dc offset" <- w221
              n94 = case shown="True" w226 {
                tunnel: [Mode."Offset" ("Enum") Mode."Process" ("Enum")] -> w224
                tunnel: w221 -> [_ w246]
                tunnel: [TRUE FALSE] -> w220
                frame False {
                }
                frame True {
                  n95 = local read "B/V (T/V)"() -> (w247:dbl)
                  n96 = local read "Gain (V/A)"() -> (w248:dbl)
                  n97 = local read "refnum out"() -> (w252:refnum<file>)
                  n98 = local read "I0 (A)"() -> (w250:dbl)
                  n99 = local read "V/I (Ohm)"() -> (w251:dbl)
                  n100 = local read "B0 (T)"() -> (w249:dbl)
                  n101 = call "File_header_diag.vi"("OFFSET"=w246, "B0"=w249, "B/V"=w247, "I0"=w250, "V/I"=w251, "Gain"=w248, "Byte Stream File in"=w252) -> ()  [unwired: 5 in]
                  n102 = local write "Offset?"(TRUE ("Offset?")) -> ()
                  n103 = Get Date/Time In Seconds() -> (seconds since 1Jan1904=→"Start time":timestamp)
                }
              }
            }
            frame "Process", Default {
              # "Converted to pA"
              # "Magnetic Field"
              # "IV converter"
              # "Elapsed Time"
              n104 = local read "Start time"() -> (w289:timestamp)
              n105 = Unbundle(w291) -> ("seconds since 1Jan1904"=w290:timestamp, "read buffer"=w284:string, "read buffer"=w271:string)
              n106 = local read "B/V (T/V)"() -> (w261:dbl)
              n107 = Fract/Exp String To Number(string=w271) -> (number=w281:dbl)  [unwired: 3 in, 1 out]
              n108 = Subtract(x=w290, y=w289) -> (x-y=w266:dbl)
              n109 = Fract/Exp String To Number(string=w284) -> (number=w285:dbl)  [unwired: 3 in, 1 out]
              n110 = Divide(x="Gain (V/A)", y=1000000000000.0) -> (x/y=w264:dbl)
              n111 = Divide(x=w285, y=w264) -> (x/y=w259:dbl)
              n112 = Subtract(x=w266, y=w265) -> (x-y=→"Time Lag":dbl)
              n113 = Build Array (concatenate)(w279, w266) -> (w288:dbl[])
              "Elapsed Time (s)" <- w288
              n114 = local read "Dc offset"() -> (w257:dbl)
              n115 = Subtract(x=w259, y=w257) -> (x-y=w258:dbl)
              "Actual Current (pA)" <- w258
              n116 = Build Array (concatenate)(w286, w258) -> (w287:dbl[])
              "Measured Current (pA)" <- w287
              n117 = local read "B0 (T)"() -> (w260:dbl)
              n118 = xnode "B(U) conversion"("V"=w281, "BpV"=w261, "B0"=w260) -> ("Result"=w280:dbl)  [unwired: 1 in, 1 out]
              "Actual B Field (T)" <- w280
              n119 = Build Array (concatenate)(w282, w280) -> (w283:dbl[])
              "Magnetic Field (T)" <- w283
              n120 = Quotient & Remainder(x=w266, y="Temp Refresh (s)") -> (floor(x/y)=w278:dbl)  [unwired: 1 out]
              n121 = Greater?(x=w278, y=w277) -> (0:w276:bool)
              "Read?" <- w276
              n122 = case shown="True" w276 {
                tunnel: [w297 w322] -> w273
                tunnel: w270 -> [w298 w321]
                tunnel: [w298 w301] -> w269
                tunnel: T5 {"Com Port"=1, "ISOBUS Address"=0, "GPIB Address"=25, "Communication"=enum."GPIB"} ("Address") -> [_ w320]
                tunnel: [w296 w316] -> w255
                frame False {
                  n123 = local read "Setpoint Temperature (K)"() -> (w296:dbl)
                  n124 = local read "Actual Temperature (K)"() -> (w297:dbl)
                }
                frame True {
                  w317 = u32 1000 ("byte count")
                  # "Temperature/Magnet read"
                  n125 = local read "Lock_in_Amplifier"() -> (w305:refnum<visa-resource-name>)
                  n126 = local read "Lake Shore"() -> (w319:refnum<visa-resource-name>)
                  n127 = local read "Magnet"() -> (w308:bool)
                  n128 = case shown="False" w308 {
                    tunnel: w320 -> [_ w326]
                    frame False {
                    }
                    frame True {
                      n129 = call "GPIB - BusCommand.vi"("Command"="R7" ("format string"), "Address"=w326) -> ("Reply"=w327:string)  [unwired: 1 out]
                      n130 = Scan From String(format string="R%f" ("remaining string"), input string=w327) -> (output 1=w325:dbl)  [unwired: 3 in, 3 out]
                      n131 = local write "Actual Field (T)"(w325) -> ()
                    }
                  }
                  n132 = VISA Write(VISA resource name=w319, write buffer="KRDG?a", error in (no error)=w321) -> (VISA resource name out=w315:refnum<visa-resource-name>, error out=w313:errorcluster)  [unwired: 1 out]
                  n133 = VISA Read(VISA resource name=w315, byte count=w317, error in (no error)=w313) -> (VISA resource name out=w314:refnum<visa-resource-name>, read buffer=w323:string, error out=w312:errorcluster)  [unwired: 1 out]
                  n134 = VISA Write(VISA resource name=w314, write buffer="SETP?a", error in (no error)=w312) -> (VISA resource name out=w310:refnum<visa-resource-name>, error out=w311:errorcluster)  [unwired: 1 out]
                  n135 = Fract/Exp String To Number(string=w323) -> (number=w322:dbl)  [unwired: 3 in, 1 out]
                  n136 = VISA Read(VISA resource name=w310, byte count=w317, error in (no error)=w311) -> (read buffer=w309:string, error out=w307:errorcluster)  [unwired: 2 out]
                  n137 = VISA Write(VISA resource name=w305, write buffer="OUTP? 3", error in (no error)=w307) -> (VISA resource name out=w304:refnum<visa-resource-name>, error out=w306:errorcluster)  [unwired: 1 out]
                  n138 = VISA Read(VISA resource name=w304, byte count=u32 1000, error in (no error)=w306) -> (read buffer=w300:string, error out=w301:errorcluster)  [unwired: 2 out]
                  n139 = Fract/Exp String To Number(string=w300) -> (number=→"LockInR":dbl)  [unwired: 3 in, 1 out]
                  n140 = Fract/Exp String To Number(string=w309) -> (number=w316:dbl)  [unwired: 3 in, 1 out]
                }
              }
              "Actual Temperature (K)" <- w273
              "Setpoint Temperature (K)" <- w255
              n141 = Build Array (concatenate)(w275, w273) -> (w274:dbl[])
              "Temperature array" <- w274
              n142 = case shown="True" "Sweep" {
                tunnel: [Mode."Plot" ("Enum") Mode."Sweep" ("Enum")] -> w272
                frame False {
                }
                frame True {
                }
              }
            }
            frame "Sweep" {
              n143 = local read "Temp/Magnetic Field"() -> (w343:bool)
              n144 = case shown="True" w343 {
                tunnel: w353 -> [w362 w419]
                tunnel: [w361 w418] -> w352
                frame False {
                  n145 = local read "Actual Field (T)"() -> (w357:dbl)
                  n146 = local read "Min Field (T)"() -> (w356:dbl)
                  n147 = local read "Max Field (T)"() -> (w363:dbl)
                  n148 = local read "Read?"() -> (w360:bool)
                  n149 = Greater Or Equal?(x=w356, y=w357) -> (x >= y?=w359:bool)
                  n150 = Compound Arithmetic op=AND(w359, w360) -> (w358:bool)
                  n151 = case shown="False" w358 {
                    tunnel: [w366 w402] -> w361
                    tunnel: w363 -> [w364 w401]
                    tunnel: w356 -> [_ w400]
                    tunnel: w357 -> [_ w398]
                    tunnel: w362 -> [w367 w397]
                    frame True {
                      # "Ramp Up"
                      n152 = case shown="True" "First?" {
                        tunnel: [TRUE ("Save") FALSE ("Save")] -> w370
                        tunnel: [w389 w393] -> w369
                        frame False {
                          n153 = local read "Counter"() -> (w392:i8)
                          n154 = local write "Actual Polarization"(0.0 ("Actual Polarization")) -> ()
                          n155 = Increment(x=w392) -> (x+1=w389:i8)
                          n156 = local write "Counter"(w389) -> ()
                        }
                        frame True {
                          n157 = local read "Counter"() -> (w393:i8)
                          n158 = local write "First?"(FALSE ("First?")) -> ()
                        }
                      }
                      "Reset" <- w370
                      n159 = local write "Read?"(FALSE ("Read?")) -> ()
                      n160 = local read "Record ALL"() -> (w365:bool)
                      n161 = case shown="True" w365 {
                        tunnel: w369 -> [_ w377]
                        tunnel: [FALSE w375] -> w368
                        frame False {
                        }
                        frame True {
                          n162 = Greater?(x=w377, y="Max Countl") -> (0:w375:bool)
                        }
                      }
                      n163 = case shown="False" w368 {
                        tunnel: w367 -> [w381 w388]
                        tunnel: [w380 w388] -> w366
                        tunnel: w364 -> [w379 _]
                        frame False {
                          n164 = local read "Magnet"() -> (w378:bool)
                          n165 = case shown="True" w378 {
                            tunnel: w381 -> [w382 w385]
                            tunnel: [w382 w384] -> w380
                            tunnel: w379 -> [_ w383]
                            frame False {
                            }
                            frame True {
                              n166 = call "Set_B.vi"("error in (no error)"=w385, "address string"="25", "Set Field (T)"=w383) -> ("error out"=w384:errorcluster)  [unwired: 8 in]
                            }
                          }
                          "Target Field" <- w379
                        }
                        frame True {
                          "New" <- TRUE
                        }
                      }
                      "Up/Down" <- FALSE ("Up/Down")
                    }
                    frame False {
                      n167 = Less Or Equal?(x=w401, y=w398) -> (x <= y?=w399:bool)
                      n168 = case shown="False" w399 {
                        tunnel: [w403 w407] -> w402
                        tunnel: w400 -> [_ w405]
                        tunnel: w397 -> [w403 w408]
                        frame False {
                        }
                        frame True {
                          # "Resetting at the end of every cycle"
                          # "Ramp Dn"
                          n169 = local write "Up/Down"(TRUE ("Up/Down")) -> ()
                          n170 = local read "Magnet"() -> (w404:bool)
                          n171 = local write "Target Field"(w405) -> ()
                          n172 = local write "Reset"(TRUE ("Reset")) -> ()
                          n173 = case shown="True" w404 {
                            tunnel: w408 -> [w410 w413]
                            tunnel: [w410 w412] -> w407
                            tunnel: w405 -> [_ w411]
                            frame False {
                            }
                            frame True {
                              n174 = call "Set_B.vi"("error in (no error)"=w413, "address string"="25", "Set Field (T)"=w411) -> ("error out"=w412:errorcluster)  [unwired: 8 in]
                            }
                          }
                        }
                      }
                      n175 = local write "Read?"(FALSE ("Read?")) -> ()
                    }
                  }
                }
                frame True {
                  n176 = local read "Setpoint Temperature (K)"() -> (w417:dbl)
                  n177 = local read "Min Temperature (K)"() -> (w416:dbl)
                  n178 = local read "Read?"() -> (w422:bool)
                  n179 = local read "Max temperature (K)"() -> (w415:dbl)
                  n180 = Equal?(x=w417, y=w416) -> (x = y?=w420:bool)
                  n181 = And(x=w420, y=w422) -> (x .and. y?=w421:bool)
                  n182 = case shown="False" w421 {
                    tunnel: [w424 w441] -> w418
                    tunnel: w415 -> [w423 w440]
                    tunnel: w416 -> [_ w439]
                    tunnel: w417 -> [_ w437]
                    tunnel: w419 -> [w425 w436]
                    frame True {
                      # "Ramp Up"
                      n183 = local read "First?"() -> (w431:bool)
                      n184 = case shown="False" w431 {
                        frame False {
                          n185 = local read "Counter"() -> (w434:i8)
                          n186 = Increment(x=w434) -> (x+1=w433:i8)
                          n187 = local write "Counter"(w433) -> ()
                        }
                        frame True {
                        }
                      }
                      n188 = local write "Read?"(FALSE ("Read?")) -> ()
                      n189 = Number To Fractional String(number=w423, precision (6)=i16 3) -> (F-format string=w428:string)  [unwired: 2 in]
                      n190 = local read "Lake Shore"() -> (w426:refnum<visa-resource-name>)
                      n191 = Concatenate Strings("SETP 1," ("write buffer"), w428) -> (w430:string)
                      n192 = VISA Write(VISA resource name=w426, write buffer=w430, error in (no error)=w425) -> (error out=w424:errorcluster)  [unwired: 2 out]
                    }
                    frame False {
                      n193 = Equal?(x=w440, y=w437) -> (x = y?=w438:bool)
                      n194 = case shown="True" w438 {
                        tunnel: [w442 w445] -> w441
                        tunnel: w439 -> [_ w444]
                        tunnel: w436 -> [w442 w446]
                        frame False {
                        }
                        frame True {
                          # "Ramp Dn"
                          n195 = local write "Up/Down"(TRUE ("Up/Down")) -> ()
                          n196 = Number To Fractional String(number=w444, precision (6)=i16 3) -> (F-format string=w448:string)  [unwired: 2 in]
                          n197 = local read "Lake Shore"() -> (w443:refnum<visa-resource-name>)
                          n198 = Concatenate Strings("SETP 1," ("write buffer"), w448) -> (w450:string)
                          n199 = VISA Write(VISA resource name=w443, write buffer=w450, error in (no error)=w446) -> (error out=w445:errorcluster)  [unwired: 2 out]
                        }
                      }
                      n200 = local write "Read?"(FALSE ("Read?")) -> ()
                    }
                  }
                }
              }
              n201 = local read "Magnet"() -> (w342:bool)
              n202 = case shown="False" w342 {
                tunnel: [Mode."StepField" ("Enum") Mode."Plot" ("Enum")] -> w344
                frame False {
                }
                frame True {
                }
              }
            }
            frame "StepField" {
              n203 = flat-sequence {
                tunnel: w453 -> [w469]
                tunnel: [w468] -> w452
                frame #0 {
                  # "Check if it is time to step Field"
                  n204 = local read "Sweep Rate (T/min)"() -> (w470:dbl)
                  n205 = local read "B/V (T/V)"() -> (w462:dbl)
                  n206 = local read "Time Lag"() -> (w466:dbl)
                  n207 = xnode "Sweep Delay"("SweepRate"=w470, "Resolution"=0.001 ("Voltage Step (V)"), "BpV"=w462) -> ("Result"=w467:dbl)  [unwired: 1 in, 1 out]
                  n208 = Divide(x=w466, y=w467) -> (x/y=w464:dbl)
                  n209 = Multiply(x=0.001 ("y"), y=w464) -> (x*y=w463:dbl)
                  "deltaUaux" <- w463
                  n210 = stacked-sequence {
                    tunnel: w469 -> [_ w494]
                    tunnel: [_ w493] -> w468
                    tunnel: w463 -> [w472 _]
                    frame #0 {
                      n211 = local read "Actual Voltage (V)"() -> (w477:dbl)
                      n212 = local read "Up/Down"() -> (w478:bool)
                      n213 = Add(x=w477, y=w472) -> (x+y=w474:dbl)
                      n214 = Subtract(x=w477, y=w472) -> (x-y=w473:dbl)
                      n215 = Select(t=w473, s=w478, f=w474) -> (s? t:f=w476:dbl)
                      "Actual Voltage (V)" <- w476
                      n216 = local read "V/I (Ohm)"() -> (w479:dbl)
                      n217 = local read "B/V (T/V)"() -> (w480:dbl)
                      n218 = xnode "AUXtoB"("BpV"=w480, "Rm"=w479, "Aux"=w476) -> ("Result"=w475:dbl)  [unwired: 1 in, 1 out]
                      n219 = local write "Actual Field (T)"(w475) -> ()
                    }
                    frame #1 {
                      n220 = local read "Actual Voltage (V)"() -> (w499:dbl)
                      n221 = local read "Lock_in_Amplifier"() -> (w495:refnum<visa-resource-name>)
                      n222 = Format Into String(w499) -> (resulting string=w498:string)  [unwired: 3 in, 1 out]
                      n223 = Concatenate Strings("AUXV 1,", w498) -> (w496:string)
                      n224 = VISA Write(VISA resource name=w495, write buffer=w496, error in (no error)=w494) -> (error out=w493:errorcluster)  [unwired: 2 out]
                    }
                  }
                }
              }
            }
            frame "Plot" {
              # "dI"
              n225 = local read "P(uC/mm^2)"() -> (w513:dbl[])
              n226 = local read "Actual Polarization"() -> (w512:dbl)
              n227 = local read "Actual Current (pA)"() -> (w514:dbl)
              n228 = local read "Time Lag"() -> (w526:dbl)
              n229 = Multiply(x=w514, y=w526) -> (x*y=w518:dbl)
              n230 = Divide(x=w518, y="Sample area (mm^2)") -> (x/y=w517:dbl)
              n231 = Add(x=w517, y=w512) -> (x+y=w516:dbl)
              "Actual Polarization" <- w516
              n232 = local read "Temp/Magnetic Field"() -> (w527:bool)
              n233 = Build Array (concatenate)(w513, w516) -> (→"P(uC/mm^2)":dbl[])
              n234 = case shown="False" w527 {
                tunnel: w524 -> [_ w587]
                tunnel: w521 -> [_ w569]
                tunnel: w516 -> [w534 w570]
                frame False {
                  # "Magnetic Field plotting"
                  n235 = local read "Up/Down"() -> (w539:bool)
                  n236 = case shown="True" w539 {
                    frame True {
                      # "Down"
                      n237 = local read "I(B) 3"() -> (w549:cluster{dbl[], dbl[]}[])
                      n238 = local read "I(B) 3"() -> (w553:cluster{dbl[], dbl[]}[])
                      n239 = Index Array(array=w549, index=1) -> (element=w547:cluster{dbl[], dbl[]})
                      n240 = Unbundle(w547) -> (w546:dbl[], w545:dbl[])
                      n241 = Index Array(array=w553, index=i8 0 ("t")) -> (element=w550:cluster{dbl[], dbl[]})
                      n242 = local read "Actual Current (pA)"() -> (w540:dbl)
                      n243 = local read "Actual B Field (T)"() -> (w542:dbl)
                      n244 = Build Array (concatenate)(w546, w542) -> (w544:dbl[])
                      n245 = Build Array (concatenate)(w545, w540) -> (w543:dbl[])
                      n246 = Bundle(w544, w543) -> (w541:cluster{dbl[], dbl[]})  [unwired: 1 in]
                      n247 = Build Array(w550, w541) -> (w551:cluster{dbl[], dbl[]}[])
                      n248 = local write "I(B) 3"(w551) -> ()
                    }
                    frame False {
                      # "Up"
                      n249 = local read "I(B) 3"() -> (w565:cluster{dbl[], dbl[]}[])
                      n250 = local read "I(B) 3"() -> (w567:cluster{dbl[], dbl[]}[])
                      n251 = Index Array(array=w565, index=0) -> (element=w563:cluster{dbl[], dbl[]})
                      n252 = Unbundle(w563) -> (w562:dbl[], w561:dbl[])
                      n253 = Index Array(array=w567, index=i8 1 ("t")) -> (element=w556:cluster{dbl[], dbl[]})
                      n254 = local read "Actual B Field (T)"() -> (w557:dbl)
                      n255 = Build Array (concatenate)(w562, w557) -> (w560:dbl[])
                      n256 = local read "Actual Current (pA)"() -> (w554:dbl)
                      n257 = Build Array (concatenate)(w561, w554) -> (w559:dbl[])
                      n258 = Bundle(w560, w559) -> (w558:cluster{dbl[], dbl[]})  [unwired: 1 in]
                      n259 = Build Array(w558, w556) -> (w555:cluster{dbl[], dbl[]}[])
                      n260 = local write "I(B) 3"(w555) -> ()
                    }
                  }
                  n261 = local read "Actual B Field (T)"() -> (w536:dbl)
                  n262 = local read "P(B)"() -> (w538:cluster{"yi":dbl[], dbl[]})
                  n263 = Unbundle(w538) -> ("yi"=w537:dbl[], w535:dbl[])
                  n264 = Build Array (concatenate)(w537, w536) -> (w533:dbl[])
                  n265 = Build Array (concatenate)(w535, w534) -> (w532:dbl[])
                  n266 = Bundle(w533, w532) -> (→"P(B)":cluster{dbl[], dbl[]})  [unwired: 1 in]
                }
                frame True {
                  # "Temperature plotting"
                  n267 = Quotient & Remainder(x=w587, y="Save Period") -> (x-y*floor(x/y)=w568:dbl)  [unwired: 1 out]
                  n268 = Greater?(x=w569, y=w568) -> (0:w585:bool)
                  n269 = local read "Actual Temperature (K)"() -> (w572:dbl)
                  n270 = local read "Actual Current (pA)"() -> (w578:dbl)
                  n271 = local read "P(T)"() -> (w574:cluster{"yi":dbl[], dbl[]})
                  n272 = local read "I(T)"() -> (w584:cluster{dbl[], dbl[]})
                  n273 = case shown="True" w585 {
                    frame False {
                    }
                    frame True {
                      n274 = local write "Reset"(TRUE) -> ()
                    }
                  }
                  n275 = Unbundle(w574) -> ("yi"=w575:dbl[], w571:dbl[])
                  n276 = Unbundle(w584) -> (w582:dbl[], w581:dbl[])
                  n277 = Build Array (concatenate)(w575, w572) -> (w576:dbl[])
                  n278 = Build Array (concatenate)(w571, w570) -> (w577:dbl[])
                  n279 = Build Array (concatenate)(w582, w572) -> (w580:dbl[])
                  n280 = Build Array (concatenate)(w581, w578) -> (w579:dbl[])
                  n281 = Bundle(w580, w579) -> (→"I(T)":cluster{dbl[], dbl[]})  [unwired: 1 in]
                  n282 = Bundle(w576, w577) -> (→"P(T)":cluster{dbl[], dbl[]})  [unwired: 1 in]
                }
              }
            }
            frame "Save" {
              n283 = local read "Reset"() -> (w589:bool)
              n284 = case shown="True" w589 {
                tunnel: w594 -> [w611 w613]
                tunnel: [w611 w616] -> w599
                tunnel: w593 -> [w610 w614]
                tunnel: [w610 w616] -> w598
                tunnel: w595 -> [w609 w615]
                tunnel: [w609 w616] -> w597
                tunnel: [w608 w616] -> w596
                tunnel: w592 -> [w608 w612]
                frame False {
                }
                frame True {
                  n285 = stacked-sequence {
                    tunnel: [_ _ w666] -> w616
                    tunnel: w615 -> [_ w655 _]
                    tunnel: w614 -> [w640 w653 _]
                    tunnel: w613 -> [w641 w654 _]
                    tunnel: w612 -> [w630 w651 _]
                    frame #0 {
                      n286 = local read "B array"() -> (w623:dbl[])
                      n287 = local read "Counter"() -> (w639:i8)
                      n288 = local read "Averaged I(B)"() -> (w643:dbl[][])
                      n289 = local read "Up/Down"() -> (w642:bool)
                      n290 = local read "Sample area (mm^2)"() -> (w619:dbl)
                      n291 = call "Average_IBP_curves.vi"("I in"=w640, "Averaged P(B) In"="Averaged P(B)", "Counter"=w639, "Averaged I(B) In"=w643, "t in"=w630, "B in"=w641, "Averaged dt in"="Averaged dt", "Up/Down"=w642, "Sample area(mm^2)"=w619, "B array"=w623) -> ("Averaged I(B) out"=w634:dbl[][], "Averaged dt Out"=w627:dbl[][], "Averaged P(B) Out"=w626:dbl[][])  [unwired: 3 in]
                      "Averaged I(B)" <- w634
                      n292 = Index Array(array=w626, index (row)=0 ("disabled index (col)")) -> (element=w624:dbl[])  [unwired: 1 in]
                      n293 = Index Array(array=w626, index (row)=1 ("disabled index (col)")) -> (element=w625:dbl[])  [unwired: 1 in]
                      n294 = local write "Averaged P(B)"(w626) -> ()
                      n295 = Index Array(array=w634, index (row)=0 ("disabled index (col)")) -> (element=w632:dbl[])  [unwired: 1 in]
                      n296 = Index Array(array=w634, index (row)=1 ("disabled index (col)")) -> (element=w631:dbl[])  [unwired: 1 in]
                      n297 = local write "Averaged dt"(w627) -> ()
                      n298 = Bundle("B array"=w623, "Averaged P(B) Out"=w624) -> (w622:T7)  [unwired: 1 in]
                      n299 = Bundle("B array"=w623, "Averaged P(B) Out"=w625) -> (w621:T7)  [unwired: 1 in]
                      n300 = Bundle("B array"=w623, "Averaged I(B) out"=w632) -> (w638:T8)  [unwired: 1 in]
                      n301 = Bundle("B array"=w623, "Averaged I(B) out"=w631) -> (w637:T8)  [unwired: 1 in]
                      n302 = Build Array(w622, w621) -> (→"P(B) /Averaged/":T9)
                      n303 = Build Array(w638, w637) -> (→"I(B) /Averaged/":T10)
                    }
                    frame #1 {
                      # "Save and Reset"
                      n304 = local read "Temp/Magnetic Field"() -> (w644:bool)
                      n305 = local read "Measurement File"() -> (w646:path)
                      n306 = local read "P(uC/mm^2)"() -> (w652:dbl[])
                      n307 = Build Array(w655, w654, w653, w651, w652) -> (w645:dbl[][])
                      n308 = case shown="False" w644 {
                        tunnel: w646 -> [_ _]
                        tunnel: w645 -> [w660 _]
                        frame False {
                          n309 = local read "Up/Down"() -> (w658:bool)
                          n310 = case shown="False" w658 {
                            tunnel: [w663 w664] -> w657
                            frame False {
                              n311 = local read "Measurement File_dn"() -> (w663:path)
                            }
                            frame True {
                              n312 = local read "Measurement File_up"() -> (w664:path)
                            }
                          }
                          n313 = call-poly <vilib>:"Write Delimited Spreadsheet.vi"("file path (dialog if empty)"=w657, "format (%.3f)"="%.5g", "2D data"=w660, "append to file? (F)"=TRUE ("transpose? (F)"), "transpose? (F)"=FALSE ("append to file? (F)")) -> ()  [unwired: 9 in, 2 out]
                        }
                        frame True {
                        }
                      }
                      n314 = case shown="False" "Reset IB?" {
                        frame False {
                        }
                        frame True {
                          n315 = local read "Up/Down"() -> (w665:bool)
                          n316 = case shown="False" w665 {
                            frame False {
                              n317 = invoke on="I(B) 3" class="XYGraph (strict)" method="Reinit To Default"() -> ()  [unwired: 3 in, 3 out]
                            }
                            frame True {
                            }
                          }
                        }
                      }
                      n318 = call-poly <vilib>:"Write Delimited Spreadsheet.vi"("file path (dialog if empty)"=w646, "format (%.3f)"="%.5g", "2D data"=w645, "append to file? (F)"=TRUE, "transpose? (F)"=TRUE) -> ()  [unwired: 9 in, 2 out]
                      n319 = local write "Reset"(FALSE ("Save")) -> ()
                    }
                    frame #2 {
                      w666 = dbl[] []
                      n320 = local write "P(uC/mm^2)"(w666) -> ()
                    }
                  }
                }
              }
              n321 = local read "New"() -> (w591:bool)
              n322 = case shown="True" w591 {
                tunnel: [Mode."Return" ("Enum") Mode."New" ("Enum")] -> w603
                tunnel: [TRUE FALSE] -> w590
                frame False {
                }
                frame True {
                }
              }
            }
            frame "New" {
              n323 = stacked-sequence {
                seq-local: [_ _ _ _ w760 _ _] -> [_ _ _ _ _ w769 _]
                seq-local: [_ _ w714 _ _ _ _] -> [_ _ _ _ w759 _ _]
                tunnel: T5 {"Com Port"=1, "ISOBUS Address"=0, "GPIB Address"=25, "Communication"=enum."GPIB"} ("Address") -> [_ _ w713 w754 _ _ _]
                tunnel: w669 -> [_ _ w715 _ _ w770 _]
                tunnel: [_ _ _ _ _ w772 _] -> w668
                tunnel: w667 -> [_ w694 _ _ _ _ _]
                frame #0 {
                  # "Save averages"
                  n324 = local read "Measurement File_average"() -> (w682:path)
                  n325 = local read "I(B) /Averaged/"() -> (w683:cluster{"B array":dbl[], dbl[]}[])
                  n326 = Index Array(array=w683, index=0) -> (element=w686:cluster{"B array":dbl[], dbl[]})
                  n327 = Index Array(array=w683, index=1) -> (element=w687:cluster{"B array":dbl[], dbl[]})
                  n328 = Unbundle(w686) -> ("B array"=w688:dbl[], w689:dbl[])
                  n329 = Unbundle(w687) -> ("B array"=w690:dbl[], w691:dbl[])
                  n330 = Build Array(w688, w689, w690, w691) -> (w692:dbl[][])
                  n331 = call-poly <vilib>:"Write Delimited Spreadsheet.vi"("file path (dialog if empty)"=w682, "format (%.3f)"="%.5g", "2D data"=w692, "append to file? (F)"=TRUE ("transpose? (F)"), "transpose? (F)"=TRUE ("append to file? (F)")) -> ()  [unwired: 9 in, 2 out]
                }
                frame #1 {
                  w700 = dbl[] []
                  w709 = dbl[] []
                  # "Reset Flags"
                  n332 = Get Date/Time In Seconds() -> (seconds since 1Jan1904=w710:timestamp)
                  n333 = local write "Up/Down"(TRUE ("Up/Down")) -> ()
                  n334 = local write "First?"(TRUE ("First?")) -> ()
                  n335 = local write "Offset?"(FALSE ("Offset?")) -> ()
                  n336 = local write "New"(FALSE ("New")) -> ()
                  n337 = local write "P(uC/mm^2)"(w709) -> ()
                  n338 = local write "Start time"(w710) -> ()
                  n339 = local write "Offset array"(w709) -> ()
                  n340 = local write "Actual Polarization"(0.0 ("Actual Polarization")) -> ()
                  n341 = local write "Up/Down"(TRUE ("Up/Down")) -> ()
                  n342 = local write "Reset"(FALSE ("Reset")) -> ()
                  n343 = local read "B array"() -> (w703:dbl[])
                  n344 = local write "Counter"(i8 0 ("Counter")) -> ()
                  n345 = invoke on="P(B)" class="XYGraph (strict)" method="Reinit To Default"() -> ()  [unwired: 3 in, 3 out]
                  n346 = invoke on="I(B) 3" class="XYGraph (strict)" method="Reinit To Default"() -> ()  [unwired: 3 in, 3 out]
                  n347 = Multiply(x=w703, y=0.0) -> (x*y=w704:dbl[])
                  n348 = Build Array(w700, w700) -> (w708:dbl[][])
                  n349 = Bundle("B array"=w703, w704) -> (w705:cluster{"B array":dbl[], dbl[]})  [unwired: 1 in]
                  n350 = local write "Averaged I(B)"(w708) -> ()
                  n351 = Build Array(w705, w705) -> (w706:cluster{"B array":dbl[], dbl[]}[])
                  n352 = local write "I(B) /Averaged/"(w706) -> ()
                  n353 = local write "Measuring"(FALSE ("Measuring")) -> ()
                  n354 = Flush Queue(queue=w694) -> (remaining elements=→"remaining elements":T1)  [unwired: 1 in, 2 out]
                }
                frame #2 {
                  # "Step"
                  n355 = local read "Sweep Rate Array"() -> (w719:dbl[])
                  n356 = local read "j"() -> (w720:i32)
                  n357 = Increment(x=w720) -> (x+1=w716:i32)
                  n358 = Array Size(array=w719) -> (size(s)=w718:i32)
                  n359 = Less?(x=w716, y=w718) -> (x < y?=w717:bool)
                  "Step Rate" <- w717
                  n360 = case shown="True" w717 {
                    tunnel: w716 -> [_ w747]
                    tunnel: w715 -> [w723 w746]
                    tunnel: [w722 w746] -> w714
                    tunnel: w713 -> [w721 _]
                    frame False {
                      # "Step Temp?"
                      n361 = local read "Temperature Array"() -> (w727:dbl[])
                      n362 = local read "i"() -> (w728:i32)
                      n363 = Increment(x=w728) -> (x+1=w725:i32)
                      n364 = local write "j"(0 ("f")) -> ()
                      n365 = Array Size(array=w727) -> (size(s)=w726:i32)
                      n366 = Less?(x=w725, y=w726) -> (x < y?=w724:bool)
                      "Step Temp" <- w724
                      n367 = case shown="False" w724 {
                        tunnel: w725 -> [_ w745]
                        tunnel: w723 -> [w733 w744]
                        tunnel: [w732 w744] -> w722
                        tunnel: w721 -> [w731 _]
                        frame False {
                          # "Heater OFF"
                          # "Finished"
                          n368 = local write "i"(0 ("i")) -> ()
                          n369 = stacked-sequence {
                            tunnel: w733 -> [w737 _ _]
                            tunnel: [w736 _ _] -> w732
                            tunnel: w731 -> [_ w741 w742]
                            frame #0 {
                              n370 = local read "Lake Shore"() -> (w738:refnum<visa-resource-name>)
                              n371 = VISA Write(VISA resource name=w738, write buffer="RANGE,1,0", error in (no error)=w737) -> (error out=w736:errorcluster)  [unwired: 2 out]
                            }
                            frame #1 {
                              n372 = call "ips_switchHeaterOff.vi"("Instrument address"=w741, "Rate"=2.0) -> ()  [unwired: 1 out]
                            }
                            frame #2 {
                              n373 = call "GPIB - BusCommand.vi"("Command"="H0", "Address"=w742) -> ()  [unwired: 2 out]
                            }
                          }
                          n374 = local write "Record ALL"(FALSE ("Record ALL")) -> ()
                          "Finished" <- TRUE
                        }
                        frame True {
                          n375 = local write "i"(w745) -> ()
                        }
                      }
                    }
                    frame True {
                      n376 = local write "j"(w747) -> ()
                    }
                  }
                }
                frame #3 {
                  # "Set rates"
                  n377 = local read "Sweep Rate Array"() -> (w753:dbl[])
                  n378 = local read "j"() -> (w752:i32)
                  n379 = local read "j"() -> (w750:i32)
                  n380 = Index Array(array=w753, index=w752) -> (element=w751:dbl)
                  n381 = Number To Fractional String(number=w751, precision (6)=i16 3) -> (F-format string=w757:string)  [unwired: 2 in]
                  n382 = Index Array(array="Max count array", index=w750) -> (element=w748:i32)
                  n383 = local write "Max Countl"(w748) -> ()
                  n384 = Concatenate Strings("T" ("format string"), w757) -> (w758:string)
                  n385 = call "GPIB - BusCommand.vi"("Command"=w758, "Address"=w754) -> ()  [unwired: 2 out]
                  n386 = local write "Sweep Rate (T/min)"(w751) -> ()
                }
                frame #4 {
                  # "Set temperature"
                  n387 = local read "Temperature Array"() -> (w763:dbl[])
                  n388 = local read "i"() -> (w762:i32)
                  n389 = Index Array(array=w763, index=w762) -> (element=w761:dbl)
                  n390 = local read "Lake Shore"() -> (w765:refnum<visa-resource-name>)
                  n391 = Number To Fractional String(number=w761, precision (6)=i16 3) -> (F-format string=w766:string)  [unwired: 2 in]
                  n392 = Concatenate Strings("SETP 1," ("write buffer"), w766) -> (w768:string)
                  n393 = VISA Write(VISA resource name=w765, write buffer=w768, error in (no error)=w759) -> (error out=w760:errorcluster)  [unwired: 2 out]
                }
                frame #5 {
                  n394 = local read "Finished"() -> (w771:bool)
                  n395 = case shown="False" w771 {
                    tunnel: [w785 w822] -> w772
                    tunnel: w770 -> [_ _]
                    tunnel: w769 -> [w782 w822]
                    frame False {
                      w780 = "_" ("string")
                      # "Wait, create Files"
                      n396 = local read "Temperature Array"() -> (w812:dbl[])
                      n397 = local read "Sweep Rate Array"() -> (w808:dbl[])
                      n398 = local read "i"() -> (w811:i32)
                      n399 = local read "j"() -> (w809:i32)
                      n400 = Index Array(array=w812, index=w811) -> (element=w810:dbl)
                      n401 = Index Array(array=w808, index=w809) -> (element=w777:dbl)
                      n402 = Round Toward -Infinity(1:w777) -> (0:w778:dbl)
                      n403 = Number To Fractional String(use system decimal point (T)=TRUE, number=w810, precision (6)=i16 1) -> (F-format string=w813:string)  [unwired: 1 in]
                      n404 = Subtract(x=w777, y=w778) -> (x-y=w779:dbl)
                      n405 = Equal To 0?(x=w779) -> (x = 0?=w776:bool)
                      n406 = Select(t=i16 0 ("precision (6)"), s=w776, f=i16 2 ("precision (6)")) -> (s? t:f=w773:i16)
                      n407 = Number To Fractional String(use system decimal point (T)=TRUE, number=w777, precision (6)=w773) -> (F-format string=w781:string)  [unwired: 1 in]
                      n408 = Concatenate Strings("Directory", "\\" ("string"), "FileName", w780, w813, "K" ("string"), w780, w781, "Tpm" ("string")) -> (w802:string)
                      n409 = Search and Replace String(replace all?=TRUE ("replace all? (F)"), input string=w802, search string=".", replace string="p" ("substring (\"\")"), error in=w782) -> (result string=w797:string, error out=w792:errorcluster)  [unwired: 3 in, 2 out]
                      n410 = local write "Step Rate"(FALSE ("Step Rate")) -> ()
                      n411 = Concatenate Strings(w797, ".txt" ("string")) -> (w796:string)
                      n412 = local read "Step Temp"() -> (w786:bool)
                      n413 = String To Path(string=w796) -> (path=w795:path)
                      n414 = Open/Create/Replace File(file path (use dialog)=w795, error in=w792, operation (0:open)=T4."open or create") -> (refnum out=w784:refnum<file>, error out=w785:errorcluster)  [unwired: 3 in, 1 out]
                      n415 = local write "refnum out"(w784) -> ()
                      n416 = Refnum to Path(1:w784) -> (0:w787:path)
                      n417 = call "Create_sweep_files.vi"("Measurement File"=w787) -> ("Path 3"=w790:path, "Path 2"=w789:path, "Path"=w788:path)  [unwired: 8 in]
                      n418 = local write "Measurement File"(w787) -> ()
                      n419 = case shown="True" w786 {
                        frame False {
                        }
                        frame True {
                          n420 = Get Date/Time In Seconds() -> (seconds since 1Jan1904=w815:timestamp)
                          n421 = local write "Step Temp"(FALSE ("Step Temp")) -> ()
                          n422 = while {
                            tunnel: w815 -> [w820]
                            stop <- w817 stop-if-true
                            n423 = Get Date/Time In Seconds() -> (seconds since 1Jan1904=w821:timestamp)
                            n424 = Subtract(x=w821, y=w820) -> (x-y=w819:dbl)
                            "Wait (s)" <- w819
                            n425 = Greater Or Equal?(x=w819, y="secs to wait") -> (x >= y?=w817:bool)
                          }
                        }
                      }
                      n426 = local write "Measurement File_dn"(w790) -> ()
                      n427 = local write "Measurement File_average"(w788) -> ()
                      n428 = local write "Measurement File_up"(w789) -> ()
                    }
                    frame True {
                    }
                  }
                }
                frame #6 {
                  n429 = local read "Finished"() -> (w823:bool)
                  n430 = case shown="True" w823 {
                    frame False {
                      n431 = local write "Measuring"(TRUE ("Measuring")) -> ()
                    }
                    frame True {
                      n432 = local write "Measure /Pause"(FALSE ("Measure /Pause")) -> ()
                    }
                  }
                }
              }
            }
            frame "Return" {
            }
          }
        }
      }
      frame Error {
        # "Return true for any case which should stop the loop."
      }
    }
  }
  n433 = case shown="True" w37 {
    frame False {
    }
    frame True {
      n434 = invoke on="P(T)" class="XYGraph (strict)" method="Reinit To Default"() -> ()  [unwired: 3 in, 3 out]
      n435 = invoke on="I(T)" class="XYGraph (strict)" method="Reinit To Default"() -> ()  [unwired: 3 in, 3 out]
    }
  }
  n436 = while {
    shift-right: [w854] -> w77
    shift-left: w57 -> [w855]
    shift-right: [w856] -> w84
    shift-left: w85 -> [w857]
    tunnel: w80 -> [w853]
    tunnel: w79 -> [w852]
    tunnel: w23 -> [w851]
    tunnel: [w845] -> _
    tunnel: w65 -> [w844]
    tunnel: w55 -> [w843]
    stop <- "stop" stop-if-true
    n437 = event shown="[6] \"Stop\": Value Change" {
      selector: _ -> [_ _ _ _ _ _ _ _ _ _ _ _ _ _ _]
      dyn-events: _ -> [_ _ _ _ _ _ _ _ _ _ _ _ _ _ _]
      timeout: 10 -> [_ _ _ _ _ _ _ _ _ _ _ _ _ _ _]
      tunnel: w857 -> [w867 w899 w909 w923 w994 w998 w1002 w1034 w1050 w1067 w1110 w1127 w1143 w1153 w1164]
      tunnel: [w866 w899 w909 w923 w994 w998 w1002 w1034 w1050 w1067 w1110 w1127 w1143 w1153 w1164] -> w856
      tunnel: w855 -> [w865 w898 w908 w921 w993 w1000 w1004 w1035 w1049 w1066 w1111 w1129 w1147 w1157 w1166]
      tunnel: [w864 w898 w908 w920 w995 w1000 w1003 _ w1049 w1066 w1111 w1128 w1146 w1156 w1165] -> w854
      tunnel: w853 -> [w863 _ _ _ _ _ _ _ _ _ _ _ _ _ _]
      tunnel: w852 -> [w862 _ _ _ _ _ _ _ _ _ _ _ _ _ _]
      tunnel: w851 -> [w861 _ _ _ _ _ _ _ _ _ _ _ _ _ _]
      tunnel: [w859 w897 w907 w922 w996 w999 w1001 w1033 w1048 w1065 w1109 w1126 w1144 w1154 _] -> w845
      tunnel: w844 -> [w859 w897 w910 w922 w996 w999 w1001 w1033 w1048 w1065 w1109 w1126 w1144 w1154 _]
      tunnel: w843 -> [_ _ _ _ _ _ _ _ _ _ _ w1130 w1145 w1158 w1163]
      tunnel: [_ _ _ _ _ _ _ w1035 _ _ _ _ _ _ _] -> _
      event Timeout {
        n438 = event-data() -> ()  [unwired: 1 in, 3 out]
        n439 = case shown="True" "Measuring" {
          tunnel: w867 -> [w869 w888]
          tunnel: [w869 w887] -> w866
          tunnel: w865 -> [w868 _]
          tunnel: [w868 w886] -> w864
          tunnel: w863 -> [_ w879]
          tunnel: w862 -> [_ w878]
          tunnel: w861 -> [_ w873]
          frame False {
          }
          frame True {
            w876 = ":FETCh? " ("data")
            w880 = u32 1000 ("byte count")
            # "Generate the data here."
            n440 = case shown="No Error" w873 {
              selector: w873 -> [w890 w891]
              tunnel: [w890 w891] -> w872
              tunnel: [w889 _] -> w871
              frame No Error {
                n441 = Get Date/Time In Seconds() -> (seconds since 1Jan1904=w889:timestamp)
              }
              frame Error {
              }
            }
            n442 = VISA Write(VISA resource name=w879, write buffer=w876, error in (no error)=w872) -> (VISA resource name out=w885:refnum<visa-resource-name>, error out=w883:errorcluster)  [unwired: 1 out]
            n443 = VISA Write(VISA resource name=w878, write buffer=w876, error in (no error)=w883) -> (VISA resource name out=w884:refnum<visa-resource-name>, error out=w882:errorcluster)  [unwired: 1 out]
            n444 = VISA Read(VISA resource name=w885, byte count=w880, error in (no error)=w882) -> (read buffer=w874:string, error out=w881:errorcluster)  [unwired: 2 out]
            n445 = VISA Read(VISA resource name=w884, byte count=w880, error in (no error)=w881) -> (read buffer=w875:string, error out=w877:errorcluster)  [unwired: 2 out]
            n446 = Bundle("seconds since 1Jan1904"=w871, "read buffer"=w874, "read buffer"=w875) -> (w870:T6)  [unwired: 1 in]
            n447 = Enqueue Element(queue=w888, element=w870, error in (no error)=w877) -> (queue out=w887:refnum<queue>, error out=w886:errorcluster)  [unwired: 1 in, 1 out]
          }
        }
      }
      event "Max Field (T)": Value Change {
        n448 = event-data() -> ()  [unwired: 1 in, 6 out]
        n449 = Divide(x="Max Field (T)", y="dB (T)") -> (x/y=w894:dbl)
        n450 = for {
          N: w894 -> [_]
          tunnel: "dB (T)" -> [w904]
          tunnel: [w901] -> w893 mode=indexing
          tunnel: "Min Field (T)" -> [w902]
          tunnel: [0.0] -> _ mode=indexing
          i -> [w905]
          n451 = Multiply(x=w905, y=w904) -> (x*y=w903:dbl)
          n452 = Add(x=w903, y=w902) -> (x+y=w901:dbl)
        }
        "B array" <- w893
      }
      event "Sweep Rate (T/min)": Value Change {
        n453 = event-data() -> ("NewVal"=w911:dbl)  [unwired: 1 in, 5 out]
        n454 = local read "Magnet"() -> (w906:bool)
        n455 = case shown="False" w906 {
          tunnel: w911 -> [_ w918]
          tunnel: w910 -> [w912 w914]
          tunnel: [w912 w913] -> w907
          frame False {
          }
          frame True {
            n456 = Number To Fractional String(number=w918, precision (6)=i16 3) -> (F-format string=w916:string)  [unwired: 2 in]
            n457 = Concatenate Strings("T" ("format string"), w916) -> (w915:string)
            n458 = call "GPIB - BusCommand.vi"("Command"=w915, "Address"=w914) -> ("Address(thru)"=w913:T5)  [unwired: 1 out]
          }
        }
      }
      event "Field To Zero": Value Change {
        n459 = event-data() -> ()  [unwired: 1 in, 6 out]
        n460 = Two Button Dialog(message="Do you want to switch off the field?", 1:"No" ("F button name (\"Cancel\")"), 2:"Yes" ("T button name (\"OK\")")) -> (T button?=w927:bool)
        n461 = case shown="True" w927 {
          tunnel: w922 -> [_ w932]
          tunnel: w921 -> [w928 w930]
          tunnel: [w928 w929] -> w920
          frame False {
          }
          frame True {
            n462 = local read "Magnet"() -> (w931:bool)
            n463 = case shown="False" w931 {
              tunnel: w932 -> [_ w984]
              tunnel: w930 -> [w935 w981]
              tunnel: [w934 w981] -> w929
              frame False {
                n464 = local read "Lock_in_Amplifier"() -> (w933:refnum<visa-resource-name>)
                n465 = stacked-sequence {
                  seq-local: [w938 _] -> [_ w950]
                  seq-local: [w936 _] -> [_ w947]
                  tunnel: w935 -> [w940 _]
                  tunnel: [_ w953] -> w934
                  tunnel: w933 -> [w937 w948]
                  frame #0 {
                    n466 = VISA Write(VISA resource name=w937, write buffer="AUXV?1", error in (no error)=w940) -> (VISA resource name out=w944:refnum<visa-resource-name>, error out=w939:errorcluster)  [unwired: 1 out]
                    n467 = VISA Read(VISA resource name=w944, byte count=u32 1000, error in (no error)=w939) -> (read buffer=w941:string, error out=w938:errorcluster)  [unwired: 2 out]
                    n468 = Fract/Exp String To Number(string=w941) -> (number=w936:dbl)  [unwired: 3 in, 1 out]
                  }
                  frame #1 {
                    w956 = 0.001 ("Voltage Step (V)")
                    n469 = local read "Sweep Rate (T/min)"() -> (w955:dbl)
                    n470 = local read "V/I (Ohm)"() -> (w952:dbl)
                    n471 = local read "B/V (T/V)"() -> (w946:dbl)
                    n472 = xnode "Sweep Delay"("SweepRate"=w955, "Resolution"=w956, "BpV"=w946) -> ("Result"=w954:dbl)  [unwired: 1 in, 1 out]
                    n473 = call "Universal_Ramping.vi"("milliseconds to wait"=w954, "Initial Voltage (V)"=w947, "error in (no error)"=w950, "Voltage Step (V)"=w956, "Final Voltage (V)"=0.0, "VISA resource name"=w948) -> ("error out"=w953:errorcluster, "Actual Voltage (V)"=w945:dbl)  [unwired: 3 in, 1 out]
                    n474 = local write "Actual Voltage (V)"(w945) -> ()
                    n475 = xnode "AUXtoB"("BpV"=w946, "Rm"=w952, "Aux"=w945) -> ("Result"=w951:dbl)  [unwired: 1 in, 1 out]
                    n476 = local write "Actual B Field (T)"(w951) -> ()
                  }
                }
              }
              frame True {
                n477 = local read "Sweep Rate (T/min)"() -> (w983:dbl)
                n478 = call "ips_switchHeaterOff.vi"("Instrument address"=w984, "Rate"=w983) -> ("B"=w982:dbl)
                n479 = local write "Actual Field (T)"(w982) -> ()
              }
            }
          }
        }
      }
      event "Go to Set": Value Change {
        n480 = event-data() -> ()  [unwired: 1 in, 6 out]
        n481 = local read "V/I (Ohm)"() -> (w991:dbl)
        n482 = local read "B/V (T/V)"() -> (w990:dbl)
        n483 = local read "Lock_in_Amplifier"() -> (w987:refnum<visa-resource-name>)
        n484 = local read "Sweep Rate (T/min)"() -> (w989:dbl)
        n485 = local read "Magnet"() -> (w992:bool)
        n486 = call "Ramp_Field.vi"("Set Field (T) in"="Set Field (T)", "Sweep Rate (T/min)"=w989, "V/I (Ohm)"=w991, "error in (no error)"=w993, "Magnet"=w992, "B/V (T/V)"=w990, "VISA Refnum in"=w987) -> ("error out"=w995:errorcluster, "Actual Voltage (V)"=w985:dbl, "Set Field (T) out"=w988:dbl)  [unwired: 2 in]
        n487 = local write "Actual B Field (T)"(w988) -> ()
        n488 = local write "Actual Voltage (V)"(w985) -> ()
      }
      event "Measure /Pause": Value Change {
        n489 = event-data() -> ("NewVal"=w997:bool)  [unwired: 1 in, 5 out]
        n490 = local write "Measuring"(w997) -> ()
      }
      event "Stop": Value Change {
        n491 = event-data() -> ()  [unwired: 1 in, 6 out]
        n492 = local read "Measuring"() -> (w1005:bool)
        n493 = case shown="True" w1005 {
          tunnel: w1004 -> [w1006 w1009]
          tunnel: [w1006 w1010] -> w1003
          frame False {
          }
          frame True {
            w1017 = FALSE ("Measuring")
            n494 = local read "SaveSweep"() -> (w1018:bool)
            n495 = local write "Measuring"(w1017) -> ()
            n496 = local write "Measure /Pause"(w1017) -> ()
            n497 = local read "Lock_in_Amplifier"() -> (w1011:refnum<visa-resource-name>)
            n498 = case shown="True" w1018 {
              frame False {
              }
              frame True {
                n499 = local read "Measurement File_average"() -> (w1029:path)
                n500 = local read "I(B) /Averaged/"() -> (w1028:cluster{"B array":dbl[], dbl[]}[])
                n501 = Index Array(array=w1028, index=0) -> (element=w1025:cluster{"B array":dbl[], dbl[]})
                n502 = Index Array(array=w1028, index=1) -> (element=w1024:cluster{"B array":dbl[], dbl[]})
                n503 = Unbundle(w1025) -> ("B array"=w1023:dbl[], w1022:dbl[])
                n504 = Unbundle(w1024) -> ("B array"=w1021:dbl[], w1020:dbl[])
                n505 = Build Array(w1023, w1022, w1021, w1020) -> (w1019:dbl[][])
                n506 = call-poly <vilib>:"Write Delimited Spreadsheet.vi"("file path (dialog if empty)"=w1029, "format (%.3f)"="%.5g", "2D data"=w1019, "append to file? (F)"=TRUE ("transpose? (F)"), "transpose? (F)"=TRUE ("append to file? (F)")) -> ()  [unwired: 9 in, 2 out]
              }
            }
            n507 = local read "V/I (Ohm)"() -> (w1015:dbl)
            n508 = local read "Sweep Rate (T/min)"() -> (w1014:dbl)
            n509 = local read "Set Field (T)"() -> (w1016:dbl)
            n510 = local read "B/V (T/V)"() -> (w1012:dbl)
            n511 = local read "Magnet"() -> (w1013:bool)
            n512 = call "Ramp_Field.vi"("Set Field (T) in"=w1016, "Sweep Rate (T/min)"=w1014, "V/I (Ohm)"=w1015, "error in (no error)"=w1009, "Magnet"=w1013, "B/V (T/V)"=w1012, "VISA Refnum in"=w1011) -> ("error out"=w1010:errorcluster, "Actual Voltage (V)"=w1007:dbl, "Set Field (T) out"=w1008:dbl)  [unwired: 2 in]
            n513 = local write "Actual B Field (T)"(w1008) -> ()
            n514 = local write "Actual Voltage (V)"(w1007) -> ()
          }
        }
      }
      event "Sweep": Value Change {
        n515 = event-data() -> ("NewVal"=w1036:bool)  [unwired: 1 in, 5 out]
        n516 = case shown="True" w1036 {
          frame False {
          }
          frame True {
            n517 = local read "Measurement File"() -> (w1037:path)
            n518 = Two Button Dialog(message="Do you want to create additional files for the sweeping measurements?" ("string"), 1:"No" ("F button name (\"Cancel\")"), 2:"Yes" ("T button name (\"OK\")")) -> (T button?=w1039:bool)
            n519 = case shown="True" w1039 {
              tunnel: w1037 -> [_ w1044]
              frame False {
                n520 = local write "SaveSweep"(FALSE ("SaveSweep")) -> ()
              }
              frame True {
                n521 = call "Create_sweep_files.vi"("Measurement File"=w1044) -> ("Path 3"=→"Measurement File_dn":path, "Path 2"=→"Measurement File_up":path, "Path"=→"Measurement File_average":path)  [unwired: 8 in]
                "SaveSweep" <- TRUE
              }
            }
          }
        }
      }
      event "Measure Noise": Value Change {
        n522 = event-data() -> ("NewVal"=w1051:bool)  [unwired: 1 in, 5 out]
        n523 = case shown="True" w1051 {
          frame False {
          }
          frame True {
            n524 = local read "Gain (V/A)"() -> (w1056:dbl)
            n525 = call "Noise_measurement.vi"("Gain (V/A)"=w1056, "Cycles"="Cycles", "Lower Cut-Off"="Cut-Off Frequency", "minimum value"="minimum value", "Filter On"="Filter On", "maximum value"="maximum value", "physical channels"="physical channels", "rate"="Rate", "samples per channel"="Samples per channel") -> ("Current (pA) Filtered"=→"Current (pA) Filtered":waveform(dbl), "PSD (pA/Hz^1/2) Peaks Removed"=→"PSD (pA/Hz^1/2) Peaks Removed":cluster{"f0":dbl, "df":dbl, "magnitude":dbl[]}, "Current (pA)"=→"Current (pA)":dbl[], "PSD (pA/Hz^1/2)"=→"PSD (pA/Hz^1/2)":cluster{"f0":dbl, "df":dbl, "magnitude":dbl[]})  [unwired: 3 in]
          }
        }
      }
      event "Calibrate": Value Change {
        n526 = event-data() -> ()  [unwired: 1 in, 6 out]
        n527 = case shown="True" "Calibrate" {
          frame False {
          }
          frame True {
            w1071 = dbl[] []
            n528 = while {
              shift-right: [w1104] -> w1069
              shift-left: dbl[][] [] -> [w1103]
              shift-right: [w1087] -> _
              shift-left: w1071 -> [w1099]
              shift-right: [w1096] -> _
              shift-left: w1071 -> [w1098]
              shift-right: [w1086] -> _
              shift-left: w1071 -> [w1097]
              shift-right: [w1078] -> _
              shift-left: 0.0 ("Set Field out") -> [w1077]
              stop <- w1100 stop-if-true
              n529 = call "Calibtarion.vi"("Dwell Time (ms)"="Dwell Time (ms)", "V array in (V)"=w1099, "I array in (A)"=w1097, "Collected array in"=w1103, "B array in (T)"=w1098, "Set Field (T)"=w1077, "dB"="dB") -> ("Best Linear Fit"=w1088:dbl[], "appended array"=→"appended array":dbl[][], "slope"=→"B/V (T/V)":dbl, "V array out (V)"=w1087:dbl[], "Boolean"=w1102:bool, "I array out (A)"=w1086:dbl[], "intercept 2"=→"I0 (A)":dbl, "Collected array out"=w1104:dbl[][], "intercept"=→"B0 (T)":dbl, "B array Out"=w1096:dbl[], "slope 2"=→"V/I (Ohm)":dbl, "Best Linear Fit 2"=w1093:dbl[], "Set Field out"=w1078:dbl)
              n530 = Bundle("I array out (A)"=w1086, "V array out (V)"=w1087) -> (w1095:T11)  [unwired: 1 in]
              n531 = Bundle("I array out (A)"=w1086, "Best Linear Fit"=w1088) -> (w1089:T12)  [unwired: 1 in]
              n532 = Bundle("V array out (V)"=w1087, "B array Out"=w1096) -> (w1091:T13)  [unwired: 1 in]
              n533 = Bundle("V array out (V)"=w1087, "Best Linear Fit 2"=w1093) -> (w1092:T14)  [unwired: 1 in]
              n534 = Or(x=w1102, y="stop 2") -> (x .or. y?=w1100:bool)
              n535 = Build Array(w1095, w1089) -> (→"V_I":T15)
              n536 = Build Array(w1091, w1092) -> (→"B_V":T16)
            }
            n537 = flat-sequence {
              tunnel: w1069 -> [w1075]
              frame #0 {
                n538 = Two Button Dialog(message="Do you want to save calibration file?") -> (T button?=w1074:bool)  [unwired: 2 in]
                n539 = case shown="True" w1074 {
                  tunnel: w1075 -> [_ w1076]
                  frame False {
                  }
                  frame True {
                    n540 = call-poly <vilib>:"Write Delimited Spreadsheet.vi"("2D data"=w1076) -> ()  [unwired: 13 in, 2 out]
                  }
                }
              }
            }
          }
        }
      }
      event "New Measurement File": Value Change {
        n541 = event-data() -> ()  [unwired: 1 in, 6 out]
        n542 = local read "Sweep"() -> (w1106:bool)
        n543 = Open/Create/Replace File(prompt="Please select measurement file\n", operation (0:open)=T4."replace or create with confirmation") -> (refnum out=w1112:refnum<file>)  [unwired: 4 in, 2 out]
        n544 = local write "refnum out"(w1112) -> ()
        n545 = Refnum to Path(1:w1112) -> (0:w1107:path)
        n546 = case shown="True" w1106 {
          tunnel: w1107 -> [_ w1115]
          frame False {
          }
          frame True {
            n547 = Two Button Dialog(message="Do you want to create additional files for the sweeping measurements?" ("string"), 1:"No" ("F button name (\"Cancel\")"), 2:"Yes" ("T button name (\"OK\")")) -> (T button?=w1117:bool)
            n548 = case shown="False" w1117 {
              tunnel: w1115 -> [_ w1125]
              frame False {
                n549 = local write "SaveSweep"(FALSE ("SaveSweep")) -> ()
              }
              frame True {
                n550 = call "Create_sweep_files.vi"("Measurement File"=w1125) -> ("Path 3"=w1122:path, "Path 2"=w1123:path, "Path"=w1124:path)  [unwired: 8 in]
                n551 = local write "Measurement File_dn"(w1122) -> ()
                n552 = local write "Measurement File_average"(w1124) -> ()
                n553 = local write "Measurement File_up"(w1123) -> ()
                n554 = local write "SaveSweep"(TRUE) -> ()
              }
            }
          }
        }
        n555 = local write "Measurement File"(w1107) -> ()
        n556 = local write "Offset?"(FALSE ("Offset?")) -> ()
        n557 = local write "First?"(TRUE ("First?")) -> ()
      }
      event "Heater On/Off": Value Change {
        n558 = event-data() -> ()  [unwired: 1 in, 6 out]
        n559 = case shown="False" "Heater On/Off" {
          tunnel: w1130 -> [w1135 w1141]
          tunnel: w1129 -> [w1133 w1142]
          tunnel: [w1132 w1140] -> w1128
          frame False {
            n560 = VISA Write(VISA resource name=w1135, write buffer="RANGE,1,0", error in (no error)=w1133) -> (error out=w1132:errorcluster)  [unwired: 2 out]
          }
          frame True {
            n561 = Number To Decimal String(number="Heater Range") -> (decimal integer string=w1138:string)  [unwired: 1 in]
            n562 = Concatenate Strings("RANGE,1," ("write buffer"), w1138) -> (w1136:string)
            n563 = VISA Write(VISA resource name=w1141, write buffer=w1136, error in (no error)=w1142) -> (error out=w1140:errorcluster)  [unwired: 2 out]
          }
        }
      }
      event "Set temperature (K)": Value Change {
        n564 = event-data() -> ()  [unwired: 1 in, 6 out]
        n565 = local read "Set temperature (K)"() -> (w1148:dbl)
        n566 = Number To Fractional String(number=w1148, precision (6)=i16 3) -> (F-format string=w1151:string)  [unwired: 2 in]
        n567 = Concatenate Strings("SETP 1," ("write buffer"), w1151) -> (w1149:string)
        n568 = VISA Write(VISA resource name=w1145, write buffer=w1149, error in (no error)=w1147) -> (error out=w1146:errorcluster)  [unwired: 2 out]
      }
      event "Temp Ramping Rate (K/min)": Value Change {
        n569 = event-data() -> ()  [unwired: 1 in, 6 out]
        n570 = local read "Temp Ramping Rate (K/min)"() -> (w1155:dbl)
        n571 = Number To Fractional String(number=w1155, precision (6)=i16 1) -> (F-format string=w1161:string)  [unwired: 2 in]
        n572 = Concatenate Strings("RAMP 1,1," ("string"), w1161) -> (w1160:string)
        n573 = VISA Write(VISA resource name=w1158, write buffer=w1160, error in (no error)=w1157) -> (error out=w1156:errorcluster)  [unwired: 2 out]
      }
      event "Heater Range": Value Change {
        n574 = event-data() -> ()  [unwired: 1 in, 6 out]
        n575 = local read "Heater On/Off"() -> (w1167:bool)
        n576 = case shown="True" w1167 {
          tunnel: w1166 -> [w1168 w1173]
          tunnel: [w1168 w1172] -> w1165
          tunnel: w1163 -> [_ w1171]
          frame False {
          }
          frame True {
            n577 = local read "Heater Range"() -> (w1169:enum16{"Off", "Low", "Medium", "High"})
            n578 = Number To Decimal String(number=w1169) -> (decimal integer string=w1175:string)  [unwired: 1 in]
            n579 = Concatenate Strings("RANGE,1," ("write buffer"), w1175) -> (w1174:string)
            n580 = VISA Write(VISA resource name=w1171, write buffer=w1174, error in (no error)=w1173) -> (error out=w1172:errorcluster)  [unwired: 2 out]
          }
        }
      }
    }
    n581 = Reciprocal(x="Sampling rate (Hz)") -> (1/x=w849:dbl)
    n582 = Multiply(x=w849, y=1000.0) -> (x*y=w847:dbl)
    n583 = Wait Until Next ms Multiple(millisecond multiple=w847) -> ()  [unwired: 1 out]
  }
  n584 = local read "Max Field (T)"() -> (w45:dbl)
  n585 = local read "Min Field (T)"() -> (w47:dbl)
  n586 = local read "dB (T)"() -> (w46:dbl)
  n587 = Divide(x=w45, y=w46) -> (x/y=w48:dbl)
  n588 = for {
    N: w48 -> [_]
    tunnel: w46 -> [w1180]
    tunnel: [w1177] -> w8 mode=indexing
    tunnel: w47 -> [w1178]
    tunnel: [0.0] -> _ mode=indexing
    i -> [w1181]
    n589 = Multiply(x=w1181, y=w1180) -> (x*y=w1179:dbl)
    n590 = Add(x=w1179, y=w1178) -> (x+y=w1177:dbl)
  }
  n591 = Multiply(x=w8, y=0.0) -> (x*y=w5:dbl[])
  n592 = Array Size(array=w5) -> (size(s)=w4:i32)
  n593 = Decrement(x=w4) -> (x-1=w3:i32)
  n594 = local write "B array"(w8) -> ()
  n595 = Array Subset(array=w5, length=w3) -> (w2:dbl[])  [unwired: 1 in]
  n596 = Build Array(w5, w5) -> (w6:dbl[][])
  n597 = local write "Averaged I(B)"(w6) -> ()
  n598 = Build Array(w2, w2) -> (w1:dbl[][])
  n599 = local write "Averaged P(B)"(w1) -> ()
  n600 = local write "Averaged dt"(w1) -> ()
  n601 = local read "Lake Shore"() -> (w58:refnum<visa-resource-name>)
  n602 = local read "IV converter"() -> (w75:refnum<visa-resource-name>)
  n603 = local read "Magnetic Field"() -> (w74:refnum<visa-resource-name>)
  n604 = VISA Close(VISA resource name=w75, error in (no error)=w77) -> (error out=w78:errorcluster)
  n605 = VISA Close(VISA resource name=w74, error in (no error)=w78) -> (error out=w76:errorcluster)
  n606 = Release Queue(queue=w84, error in (no error)=w76) -> (error out=w71:errorcluster)  [unwired: 1 in, 2 out]
  n607 = Merge Errors(w71, w70) -> (w72:errorcluster)
  n608 = VISA Close(VISA resource name=w58, error in (no error)=w72) -> (error out=w69:errorcluster)
  n609 = local read "refnum out"() -> (w67:refnum<file>)
  n610 = Close File(refnum=w67, error in=w69) -> (error out=w68:errorcluster)  [unwired: 1 out]
  n611 = call <vilib>:"Simple Error Handler.vi"("error in (no error)"=w68) -> ()  [unwired: 4 in, 5 out]
  "i" <- w38
  "j" <- w38
